vi "sub_peltier 1 control new.vi"(0 "Save File":path, 1 "Save Data to File":bool caption="Save?", 2 "Sample Rate (s)":i16=1, 9 "COM":i16, 12 "Array #":i32, 13 "Control Settings":T1={"Control Sensor Offset"=0.0, "Set Limit Low"=-20.0, "Set Limit High"=100.0, "Derivative Gain"=0.0, "Integral Gain"=0.0, "Proportional Bandwidth"=50.0}) -> ()   [LabVIEW 2021]
uses:
  <vilib>/Instr/_visa.llb/VISA Find Search Mode.ctl
  <vilib>/Utility/error.llb/DialogType.ctl
  globalvariables.vi
  <vilib>/Utility/file.llb/Write Delimited Spreadsheet (string).vi
  <vilib>/Utility/file.llb/Write Delimited Spreadsheet (DBL).vi
panel:
  in  "Controller Settings":enum32{"Page 1"}(tab)
  in  "Alarm Settings":enum32{"Page 1"}(tab)
  in  "Shutdown Output w/ Alarm 2":bool
  in  "Clear Alarm Latch":bool
  in  "Shutdown Output w/ Alarm 1":bool
  in  "Alarm 2 Deadband":dbl
  in  "Alarm 2 Low":dbl
  in  "Alarm 2 High":dbl=60.0
  in  "Alarm 1 Deadband":dbl
  in  "Alarm 1 Low":dbl
  in  "Alarm 1 High":dbl=60.0
  in  "Alarm Latch":T2(radio)
  out "Alarm":bool
  in  "Graph Data":enum32{"Tab 1"}(tab)
  out "Elapsed Time":dbl=-3262346310.140625
  out "Start Sample Time":timestamp=timestamp(3262346310.140625 s since 1904-01-01)
  out "Sample in Time":timestamp
  out "Set Temperature":dbl
  out "Input 2 Sensor":dbl
  out "Control Sensor":dbl
  in  "Misc Settings":enum32{"Page 1"}(tab)
  in  "Analog Output Multiplier":dbl=1.0
  in  "Sensor Type":enum32{"15K", "10K"}(radio)=enum."10K"
  in  "Output Polarity":enum32{"Cool", "Heat "}(radio)
  in  "EEPROM Write Enable":bool
  in  "Temperature 2 Display":T3(radio)=enum."Radio Selection 3"
  out "Firmware Version":string
  out "CRC Error":bool
  out "error out":errorcluster
  out "Reading Configuration":sgl
  in  "Display":enum32{"Page 1"}(tab)
  out "Power":i16(slide) scale=0.0..100.0
  out "Strip Chart":T4(graph)
  out "Sampling":bool
  in  "Run Peltier":bool
  # "%"
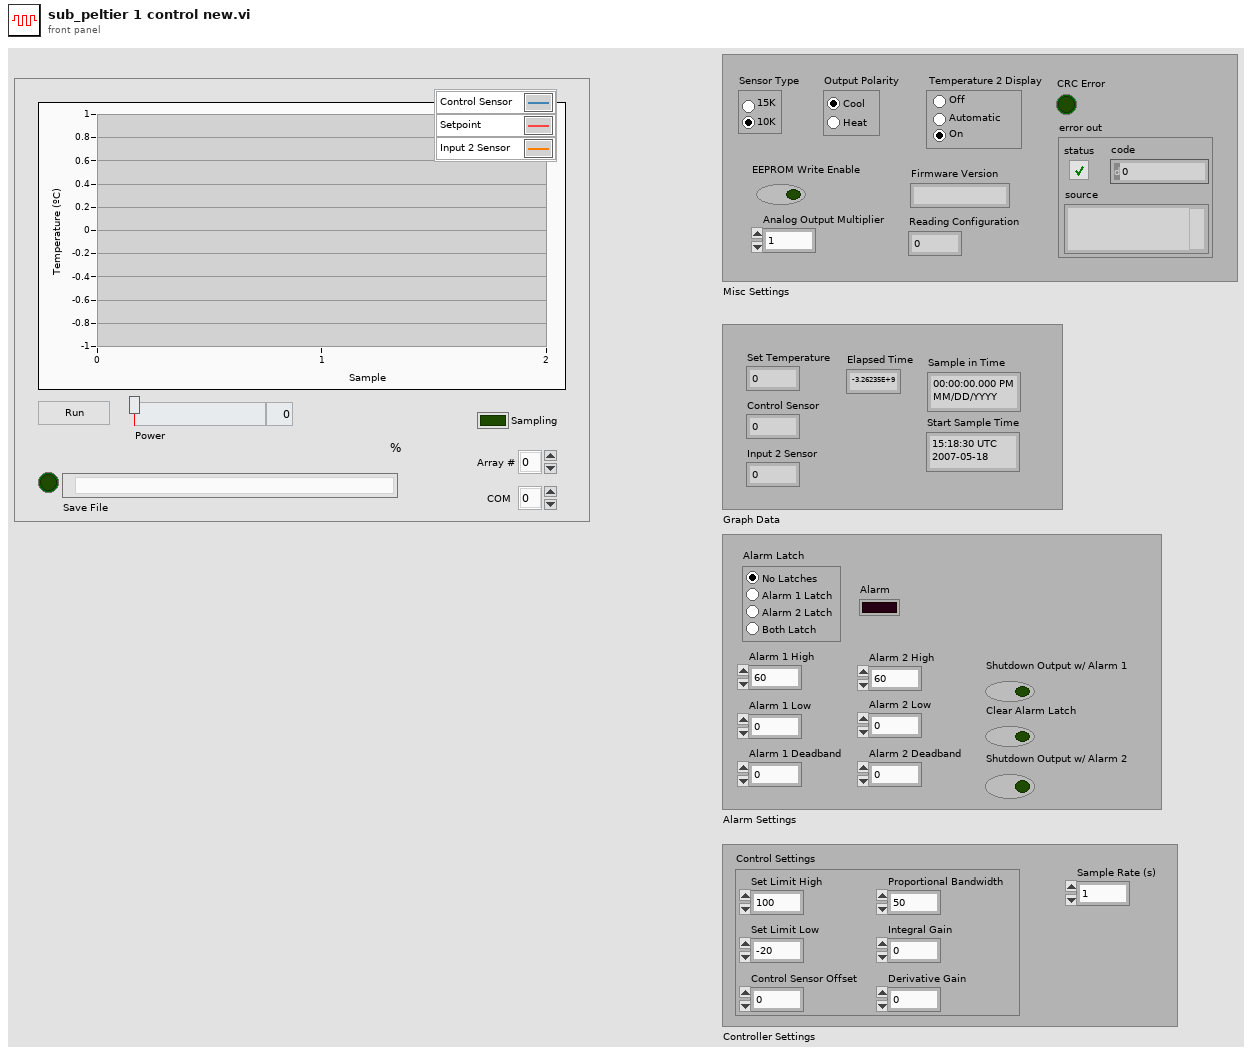
[diagram p1: front panel]
types:
  T1 = cluster{"Control Sensor Offset":dbl, "Set Limit Low":dbl, "Set Limit High":dbl, "Derivative Gain":dbl, "Integral Gain":dbl, "Proportional Bandwidth":dbl}
  T2 = enum32{"Radio Selection 1", "Radio Selection 2", "Radio Selection 3", "Radio Selection 4"}
  T3 = enum32{"Radio Selection 1", "Radio Selection 2", "Radio Selection 3"}
  T4 = cluster{"TEMPERATURE":dbl, "Value":dbl, "Value 2":dbl}
  T5 = cluster{"Read Model":bool, "Read Settings":bool, "End":bool, "CRC Error":bool, "Final Loop":bool}
  T6 = typedef "VISA Find Search Mode.ctl" = u32
  T7 = cluster{"TEMPERATURE":dbl, "Value":dbl, "Value 2":dbl}[]
  T8 = cluster{"SET POINT":dbl, "SET POINT":dbl, "SET POINT":dbl}
  T9 = typedef "DialogType.ctl" = u16
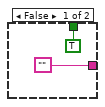
[diagram p2: hidden frame]
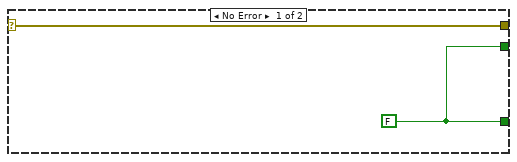
[diagram p3: hidden frame]
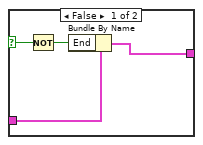
[diagram p11: hidden frame]
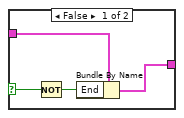
[diagram p13: hidden frame]
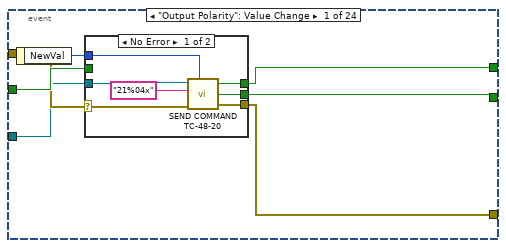
[diagram p14: hidden frame]
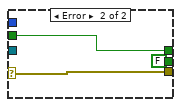
[diagram p15: hidden frame]
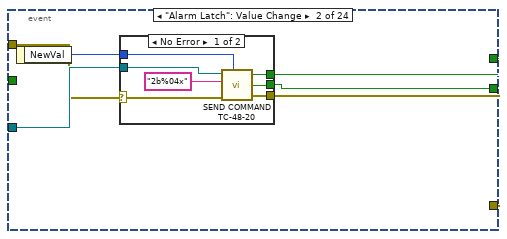
[diagram p16: hidden frame]
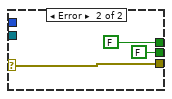
[diagram p17: hidden frame]
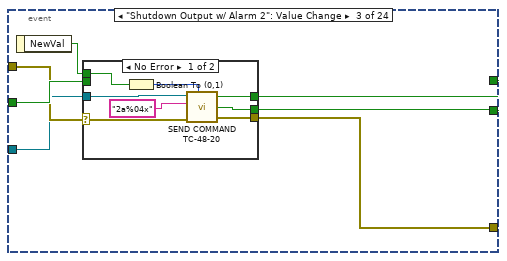
[diagram p18: hidden frame]
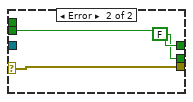
[diagram p19: hidden frame]
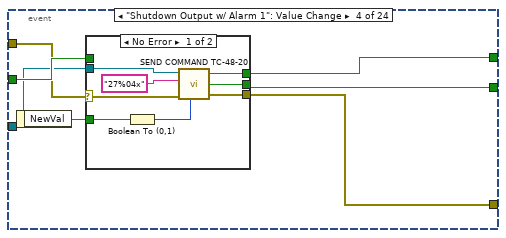
[diagram p20: hidden frame]
diagram:
  w1 = FALSE  # Final Loop
  w2 = FALSE  # CRC Error
  w3 = FALSE  # End
  w5 = TRUE  # Read Settings
  w6 = TRUE  # Read Model
  # "Connect to Peltier Controller"
  # "CHECK CONTROLS"
  n1 = Bundle("Read Model"=w6, "Read Settings"=w5, "End"=w3, "CRC Error"=w2, "Final Loop"=w1) -> (w4:T5)  [unwired: 1 in]
  n2 = while {
    tunnel: [w35] -> w10
    tunnel: [w30] -> w9
    tunnel: errorcluster {"status"=FALSE, "code"=0, "source"=""} ("Startup error in (no error)") -> [w34]
    tunnel: w4 -> [w28]
    tunnel: [w25] -> w8
    stop <- w29 continue-if-true
    w22 = u16 0 items=["None", "XON/XOFF", "RTS/CTS", "XON/XOFF & RTS/CTS", "DTR/DSR", "XON/XOFF & DTR/DSR"] ("Serial Settings:Flow Control")
    w18 = u16 0 items=["None", "Odd", "Even", "Mark", "Space"] ("Serial Settings:Parity")
    w23 = T6 4 items=["Canonical Names Only"=0, "Aliases Only"=1, "Include Matching Aliases"=2, "Include All Aliases"=4] ("Search Mode")
    n3 = Greater Than 0?(x="COM") -> (x > 0?=w13:bool)
    n4 = case shown="True" w13 {
      tunnel: "COM" -> [_ w44]
      tunnel: ["" w41] -> w11
      tunnel: [TRUE FALSE] -> w27
      frame False {
      }
      frame True {
        n5 = Number To Decimal String(number=w44) -> (decimal integer string=w42:string)  [unwired: 1 in]
        n6 = Concatenate Strings("COM", w42) -> (w41:string)
      }
    }
    n7 = property on="Firmware Version" class="Str"("Value"="") -> ()  [unwired: 2 in, 2 out]
    n8 = VISA Find Resource(8:w34, 10:w23) -> (0:w17:errorcluster)  [unwired: 1 in, 2 out]
    n9 = Coerce To Type(0:w11, 1:refnum<visa-resource-name> refnum ("SELECT PORT")) -> (2:w14:refnum<visa-resource-name>)
    n10 = property class="Instr" props=["Baud", "Data Bits", "Parity", "Stop Bits", "Flow Cntrl", "Rsrc Name", "Is Connected"](reference=w14, error in=w17, "Baud"=u32 115200 ("Numeric 6"), "Data Bits"=u16 8, "Parity"=w18, "Stop Bits"=u16 10, "Flow Cntrl"=w22) -> (reference out=w32:refnum<visa-resource-name>, error out=w33:errorcluster)  [unwired: 2 out]
    n11 = VISA Set I/O Buffer Size(VISA resource name=w32, error in (no error)=w33) -> (VISA resource name out=w36:refnum<visa-resource-name>, error out=w37:errorcluster)  [unwired: 2 in]
    n12 = VISA Flush I/O Buffer(VISA resource name=w36, error in (no error)=w37) -> (VISA resource name out=w35:refnum<visa-resource-name>, error out=w31:errorcluster)  [unwired: 1 in]
    n13 = case shown="Error" w31 {
      selector: w31 -> [w46 w50]
      tunnel: [w46 w50] -> w30
      tunnel: [w45 w48] -> w29
      tunnel: [w45 w47] -> w26
      frame No Error {
        w45 = FALSE
      }
      frame Error {
        n14 = Two Button Dialog(message=" Unable to communicate with controller (Error 1), check:\n• Controller is ON and correctly wired\n• Correct communications port is selected\n• Another program is not using the communications port ", 1:"EXIT" ("F button name (\"Cancel\")"), 2:"RESTART" ("T button name (\"OK\")")) -> (T button?=w49:bool)
        n15 = case shown="True" w49 {
          selector: w49 -> [w54 w55]
          tunnel: [w54 w55] -> w48
          frame False {
          }
          frame True {
            n16 = Wait (ms)(milliseconds to wait=u32 5000) -> ()  [unwired: 1 out]
          }
        }
        n17 = Not(x=w48) -> (.not. x?=w47:bool)
      }
    }
    n18 = Or(x=w27, y=w26) -> (x .or. y?=w24:bool)
    n19 = Bundle By Name(cluster=w28, "End"=w24) -> (w25:T5)
  }
  n20 = while {
    shift-right: [w64] -> _
    shift-left: w8 -> [w74]
    tunnel: w10 -> [w91]
    tunnel: w9 -> [w80]
    i -> [w65]
    stop <- w63 stop-if-true
    n21 = global read "globalvariables.vi" "Peltier Update"() -> (w78:bool[])
    n22 = property on="Array #" class="DigNum (strict)"() -> ("Value"=w76:i32)  [unwired: 2 in, 2 out]
    n23 = Bundle By Name(cluster=w74, "CRC Error"=FALSE) -> (w75:T5)
    n24 = Index Array(array=w78, index=w76) -> (element=w77:bool)
    n25 = case shown="True" w77 {
      tunnel: w75 -> [w105 w107]
      tunnel: [w105 w106] -> w60
      frame False {
      }
      frame True {
        n26 = global read "globalvariables.vi" "Peltier Set Temp"() -> (w115:dbl[])
        n27 = global read "globalvariables.vi" "Peltier Update"() -> (w113:bool[])
        n28 = global read "globalvariables.vi" "Peltier Stop"() -> (w108:bool)
        n29 = global read "globalvariables.vi" "Peltier Save"() -> (w109:bool)
        n30 = property on="Array #" class="DigNum (strict)"() -> ("Value"=w112:i32)  [unwired: 2 in, 2 out]
        n31 = case shown="True" w108 {
          selector: w108 -> [_ w118]
          tunnel: w107 -> [w116 w120]
          tunnel: [w116 w119] -> w106
          frame False {
          }
          frame True {
            n32 = Bundle By Name(cluster=w120, "End"=w118) -> (w119:T5)
            n33 = property on="Run Peltier" class="Bool (strict)"("Value"=FALSE ("Run Peltier")) -> ()  [unwired: 2 in, 2 out]
          }
        }
        n34 = property on="Save Data to File" class="Bool (strict)"("Value"=w109) -> ()  [unwired: 2 in, 2 out]
        n35 = Index Array(array=w115, index=w112) -> (element=w114:dbl)
        n36 = Replace Array Subset(array=w113, new element=FALSE ("Is Peltier Command Ready?"), index=w112) -> (w110:bool[])
        n37 = property on="Set Temperature" class="DigNum (strict)"("Val(Sgnl)"=w114) -> ()  [unwired: 2 in, 2 out]
        n38 = global write "globalvariables.vi" "Peltier Update"(w110) -> ()
      }
    }
    n39 = flat-sequence {
      tunnel: [w1168] -> w90
      tunnel: [w1167] -> w89
      tunnel: [w1166] -> w88
      tunnel: w60 -> [w1165]
      tunnel: w91 -> [w1164]
      tunnel: w80 -> [w1163]
      tunnel: w90 -> [w1288]
      tunnel: w89 -> [w1292]
      tunnel: w88 -> [w1291]
      tunnel: [w1290] -> w83
      tunnel: [w1289] -> w82
      tunnel: [w1287] -> w85
      frame #0 {
        n40 = case shown="No Error" w1163 {
          selector: w1163 -> [w1171 w1286]
          tunnel: [w1175 w1286] -> w1168
          tunnel: [w1174 w1285] -> w1167
          tunnel: [w1173 w1284] -> w1166
          tunnel: w1164 -> [w1172 w1285]
          tunnel: w1165 -> [w1170 w1284]
          frame No Error {
            n41 = Unbundle By Name(w1170) -> ("Read Model"=w1169:bool)
            n42 = case shown="True" w1169 {
              tunnel: [w1176 w1180] -> w1175
              tunnel: [w1177 w1182] -> w1174
              tunnel: w1170 -> [w1178 w1184]
              tunnel: [w1178 w1183] -> w1173
              tunnel: w1172 -> [w1177 w1182]
              tunnel: w1171 -> [w1176 w1179]
              frame False {
              }
              frame True {
                n43 = while {
                  tunnel: w1184 -> [w1188]
                  tunnel: [w1202] -> w1183
                  tunnel: w1182 -> [w1193]
                  tunnel: [w1194] -> w1180
                  tunnel: w1179 -> [w1190]
                  i -> [w1198]
                  stop <- w1196 stop-if-true
                  n44 = Greater Or Equal?(x=w1198, y=3) -> (x >= y?=w1197:bool)
                  n45 = call "QUERY MODEL9613.vi"("Communications Port"=w1193) -> ("error out"=w1191:errorcluster, "CRC ERROR"=w1186:bool, "CONTROLLER MODEL"=w1195:string)  [unwired: 3 in]
                  n46 = case shown="True" w1186 {
                    selector: w1186 -> [_ w1205]
                    tunnel: [w1203 w1206] -> w1187
                    tunnel: w1188 -> [w1203 w1204]
                    frame False {
                    }
                    frame True {
                      n47 = Bundle By Name(cluster=w1204, "CRC Error"=w1205) -> (w1206:T5)
                    }
                  }
                  n48 = case shown="True" w1197 {
                    tunnel: w1187 -> [w1208 w1212]
                    tunnel: [w1208 w1211] -> w1189
                    tunnel: [FALSE ("true") w1209] -> w1185
                    frame False {
                    }
                    frame True {
                      n49 = One Button Dialog(message="Commuincation Error") -> (true=w1209:bool)  [unwired: 1 in]
                      n50 = Bundle By Name(cluster=w1212, "End"=w1209) -> (w1211:T5)
                    }
                  }
                  n51 = Wait Until Next ms Multiple(millisecond multiple=u32 120) -> ()  [unwired: 1 out]
                  n52 = Equal?(x=w1195, y="9613") -> (x = y?=w1192:bool)
                  n53 = Merge Errors(w1190, w1191) -> (w1194:errorcluster)
                  n54 = Compound Arithmetic op=OR(w1192, w1186, w1185) -> (w1196:bool)
                  n55 = case shown="True" w1192 {
                    tunnel: [w1216 w1224] -> w1202
                    tunnel: w1193 -> [_ w1222]
                    tunnel: w1189 -> [w1213 w1218]
                    frame False {
                      n56 = Bundle By Name(cluster=w1213, "Read Model"=TRUE, "Read Settings"=FALSE) -> (w1216:T5)
                    }
                    frame True {
                      n57 = call "QUERY FIRMWARE VERSION M9613.vi"("Communications Port"=w1222) -> ("error out"=w1221:errorcluster, "VERSION NUMBER"=w1220:u32)  [unwired: 8 in, 1 out]
                      n58 = Bundle By Name(cluster=w1218, "Read Model"=FALSE) -> (w1224:T5)
                      n59 = case shown="No Error" w1221 {
                        tunnel: w1220 -> [w1227 _]
                        tunnel: [w1226 ""] -> w1219
                        tunnel: [w1225 2] -> w1217
                        frame No Error {
                          n60 = case shown="0, Default" w1227 {
                            tunnel: ["B" "C" "D" "E" "F" "G" "H" "I" "J" "K" "L" "M" "N" "O" "P" "Q" "R" "S" "T" "U" "V" "W" "X" "Y" "Z" "" "A"] -> w1226
                            tunnel: [2 2 2 2 2 2 0 0 0 0 0 0 0 0 0 0 0 0 0 0 0 0 0 0 0 2 2] -> w1225
                            frame 2 {
                            }
                            frame 3 {
                            }
                            frame 4 {
                            }
                            frame 5 {
                            }
                            frame 6 {
                            }
                            frame 7 {
                            }
                            frame 8 {
                            }
                            frame 9 {
                            }
                            frame 10 {
                            }
                            frame 11 {
                            }
                            frame 12 {
                            }
                            frame 13 {
                            }
                            frame 14 {
                            }
                            frame 15 {
                            }
                            frame 16 {
                            }
                            frame 17 {
                            }
                            frame 18 {
                            }
                            frame 19 {
                            }
                            frame 20 {
                            }
                            frame 21 {
                            }
                            frame 22 {
                            }
                            frame 23 {
                            }
                            frame 24 {
                            }
                            frame 25 {
                            }
                            frame 26 {
                            }
                            frame 0, Default {
                            }
                            frame 1 {
                            }
                          }
                        }
                        frame Error {
                        }
                      }
                      "Firmware Version" <- w1219
                      n61 = property on="EEPROM Write Enable" class="Bool (strict)"("Disabled"=w1217) -> ()  [unwired: 2 in, 2 out]
                    }
                  }
                }
                n62 = property on="Strip Chart" class="WFChart (strict)"("History Data"=T7 []) -> ()  [unwired: 2 in, 2 out]
              }
            }
          }
          frame Error {
          }
        }
      }
      frame #1 {
        n63 = case shown="No Error" w1288 {
          selector: w1288 -> [w1295 w1494]
          tunnel: w1292 -> [w1299 w1495]
          tunnel: w1291 -> [w1293 w1498]
          tunnel: [w1298 w1497] -> w1290
          tunnel: [w1297 w1494] -> w1289
          tunnel: [w1296 w1495] -> w1287
          frame No Error {
            n64 = Unbundle By Name(w1293) -> ("Read Settings"=w1294:bool)
            n65 = case shown="True" w1294 {
              tunnel: w1295 -> [w1302 w1312]
              tunnel: w1299 -> [w1300 w1309]
              tunnel: w1293 -> [w1303 w1306]
              tunnel: [w1303 w1311] -> w1298
              tunnel: [w1302 w1310] -> w1297
              tunnel: [w1300 w1308] -> w1296
              frame False {
                n66 = property on="Reading Configuration" class="DigNum (strict)"("Value"=0) -> ()  [unwired: 2 in, 2 out]
              }
              frame True {
                n67 = for {
                  N: 21 -> [_]
                  tunnel: w1309 -> [w1322]
                  tunnel: w1312 -> [w1328]
                  tunnel: [w1321] -> w1310
                  tunnel: [w1322] -> w1308
                  tunnel: w1306 -> [w1318]
                  tunnel: [w1315] -> w1305
                  i -> [w1313]
                  n68 = Divide(x=w1313, y=21) -> (x/y=w1327:dbl)
                  n69 = case shown="8" w1313 {
                    tunnel: w1322 -> [w1343 w1348 w1356 w1362 w1369 w1373 w1383 w1391 w1407 w1412 w1419 w1425 w1433 w1443 w1455 w1459 w1467 w1472 w1479 w1487 w1491]
                    tunnel: w1328 -> [w1339 w1347 w1353 w1360 w1368 w1372 w1382 w1386 w1406 w1410 w1416 w1422 w1428 w1442 w1454 w1461 w1465 w1473 w1478 w1486 w1492]
                    tunnel: [w1342 _ _ _ w1365 _ _ _ _ _ _ _ _ _ _ _ _ _ _ _ _] -> w1319
                    tunnel: [FALSE ("CRC") w1344 w1351 w1358 FALSE ("CRC") w1370 w1377 w1385 w1395 w1408 w1415 w1421 w1426 w1436 w1448 w1457 w1463 w1468 w1474 w1480 w1489] -> w1317
                    tunnel: [w1341 w1346 w1355 w1361 w1367 w1374 w1381 w1390 w1400 w1411 w1418 w1424 w1432 w1440 w1452 w1460 w1466 w1470 w1477 w1485 w1493] -> w1323
                    tunnel: [w1338 w1345 w1352 w1357 w1364 w1371 w1376 w1384 w1396 w1409 w1414 w1420 w1427 w1437 w1449 w1456 w1462 w1469 w1475 w1481 w1488] -> w1316
                    frame 0, Default {
                      n70 = property on="Power" class="Slide (strict)"() -> ("Value"=w1342:i16)  [unwired: 2 in, 2 out]
                      n71 = call "QUERY INPUT 1 M9613.vi"("Communications Port"=w1343, "error in"=w1339) -> ("CRC ERROR"=w1338:bool, "TEMPERATURE"=w1340:dbl, "error out"=w1341:errorcluster)
                      n72 = property on="Control Sensor" class="DigNum (strict)"("Value"=w1340) -> ()  [unwired: 2 in, 2 out]
                    }
                    frame 1 {
                      n73 = call "QUERY ALARMS M9613.vi"("Communications Port"=w1348, "error in"=w1347) -> ("CRC ERROR"=w1345:bool, "End"=w1344:bool, "ALARM VALUE"=w1349:dbl, "error out"=w1346:errorcluster)
                      n74 = Not Equal To 0?(x=w1349) -> (x != 0?=→"Alarm":bool)
                    }
                    frame 2 {
                      n75 = call "QUERY CONTROL MODE M9613.vi"("Communications Port"=w1356, "error in"=w1353) -> ("CRC ERROR"=w1352:bool, "End"=w1351:bool, "CONTROL MODE"=w1354:dbl, "error out"=w1355:errorcluster)
                      n76 = property on="Output Polarity" class="RadioBtnsControl (strict)"("Value"=w1354) -> ()  [unwired: 2 in, 2 out]
                    }
                    frame 3 {
                      n77 = call "QUERY ALARM LATCH SETTING M9613.vi"("Communications Port"=w1362, "error in"=w1360) -> ("CRC ERROR"=w1357:bool, "End"=w1358:bool, "ALARM LATCH SETTING"=w1359:dbl, "error out"=w1361:errorcluster)
                      n78 = property on="Alarm Latch" class="RadioBtnsControl (strict)"("Value"=w1359) -> ()  [unwired: 2 in, 2 out]
                    }
                    frame 4 {
                      n79 = call "QUERY POWER OUT M9613.vi"("Communications Port"=w1369, "error in"=w1368) -> ("CRC ERROR"=w1364:bool, "POWER OUT, %"=w1366:dbl, "error out"=w1367:errorcluster)
                      n80 = To Word Integer(number=w1366) -> (16bit integer=w1365:i16)
                    }
                    frame 5 {
                      n81 = call "QUERY SETPOINT M9613.vi"("Communications Port"=w1373, "error in"=w1372) -> ("CRC ERROR"=w1371:bool, "End"=w1370:bool, "SET POINT"=w1375:dbl, "error out"=w1374:errorcluster)
                      n82 = property on="Set Temperature" class="DigNum (strict)"("Value"=w1375) -> ()  [unwired: 2 in, 2 out]
                    }
                    frame 6 {
                      n83 = call "QUERY ALARM 2 STATUS M9613.vi"("Communications Port"=w1383, "error in"=w1382) -> ("CRC ERROR"=w1376:bool, "End"=w1377:bool, "ALARM 2 OUTPUT STATUS"=w1378:dbl, "error out"=w1381:errorcluster)
                      n84 = Number To Boolean Array(number=w1378) -> (Boolean array=w1380:bool[])
                      n85 = Or Array Elements(Boolean array=w1380) -> (logical OR=w1379:bool)
                      n86 = property on="Shutdown Output w/ Alarm 2" class="Bool (strict)"("Value"=w1379) -> ()  [unwired: 2 in, 2 out]
                    }
                    frame 7 {
                      n87 = call "QUERY ALARM 1 STATUS M9613.vi"("Communications Port"=w1391, "error in"=w1386) -> ("CRC ERROR"=w1384:bool, "End"=w1385:bool, "ALARM 2 OUTPUT STATUS"=w1389:dbl, "error out"=w1390:errorcluster)
                      n88 = Number To Boolean Array(number=w1389) -> (Boolean array=w1388:bool[])
                      n89 = Or Array Elements(Boolean array=w1388) -> (logical OR=w1387:bool)
                      n90 = property on="Shutdown Output w/ Alarm 1" class="Bool (strict)"("Value"=w1387) -> ()  [unwired: 2 in, 2 out]
                    }
                    frame 8 {
                      n91 = call "QUERY PROPORTIONAL BW M9613.vi"("Communications Port"=w1407, "error in"=w1406) -> ("CRC ERROR"=w1399:bool, "End"=w1394:bool, "PROPOTIONAL BW"=w1403:dbl, "error out"=w1402:errorcluster)
                      n92 = call "QUERY INTEGRAL GAIN M9613.vi"("Communications Port"=w1407, "error in"=w1402) -> ("CRC ERROR"=w1398:bool, "End"=w1393:bool, "INTEGRAL GAIN"=w1404:dbl, "error out"=w1401:errorcluster)
                      n93 = call "QUERY DERIVATIVE GAIN M9613.vi"("Communications Port"=w1407, "error in"=w1401) -> ("CRC ERROR"=w1397:bool, "End"=w1392:bool, "DERIVATIVE GAIN"=w1405:dbl, "error out"=w1400:errorcluster)
                      n94 = property on="Proportional Bandwidth" class="DigNum (strict)"("Value"=w1403) -> ()  [unwired: 2 in, 2 out]
                      n95 = property on="Integral Gain" class="DigNum (strict)"("Value"=w1404) -> ()  [unwired: 2 in, 2 out]
                      n96 = property on="Derivative Gain" class="DigNum (strict)"("Value"=w1405) -> ()  [unwired: 2 in, 2 out]
                      n97 = Compound Arithmetic op=OR(w1399, w1398, w1397) -> (w1396:bool)
                      n98 = Compound Arithmetic op=OR(w1394, w1393, w1392) -> (w1395:bool)
                    }
                    frame 9 {
                      n99 = call "INPUT 1 SENSOR OFFSET M9613.vi"("Communications Port"=w1412, "error in"=w1410) -> ("CRC ERROR"=w1409:bool, "End"=w1408:bool, "INPUT 1 SENSOR OFFSET"=w1413:dbl, "error out"=w1411:errorcluster)
                      n100 = property on="Control Sensor Offset" class="DigNum (strict)"("Value"=w1413) -> ()  [unwired: 2 in, 2 out]
                    }
                    frame 10 {
                      n101 = call "QUERY ALARM LATCH SETTING M9613.vi"("Communications Port"=w1419, "error in"=w1416) -> ("CRC ERROR"=w1414:bool, "End"=w1415:bool, "ALARM LATCH SETTING"=w1417:dbl, "error out"=w1418:errorcluster)
                      n102 = property on="Alarm Latch" class="RadioBtnsControl (strict)"("Value"=w1417) -> ()  [unwired: 2 in, 2 out]
                    }
                    frame 11 {
                      n103 = call "QUERY SENSOR TYPE M9613.vi"("Communications Port"=w1425, "error in"=w1422) -> ("CRC ERROR"=w1420:bool, "End"=w1421:bool, "SENSOR TYPE"=w1423:dbl, "error out"=w1424:errorcluster)
                      n104 = property on="Sensor Type" class="RadioBtnsControl (strict)"("Value"=w1423) -> ()  [unwired: 2 in, 2 out]
                    }
                    frame 12 {
                      n105 = call "QUERY ALARM 1 DEADBAND M9613.vi"("Communications Port"=w1433, "error in"=w1428) -> ("CRC ERROR"=w1427:bool, "End"=w1426:bool, "ALARM 1 DEADBAND"=w1430:dbl, "error out"=w1432:errorcluster)
                      n106 = Divide(x=w1430, y=10.0) -> (x/y=w1431:dbl)
                      n107 = property on="Alarm 1 Deadband" class="DigNum (strict)"("Value"=w1431) -> ()  [unwired: 2 in, 2 out]
                    }
                    frame 13 {
                      n108 = call "QUERY HIGH ALARM SET POINT M9613.vi"("Communications Port"=w1443, "error in"=w1442) -> ("CRC ERROR"=w1435:bool, "HIGH ALARM SETPOINT INPUT 1"=w1438:dbl, "error out"=w1441:errorcluster)
                      n109 = call "QUERY LOW ALARM SET POINT M9613.vi"("Communications Port"=w1443, "error in"=w1441) -> ("CRC ERROR"=w1434:bool, "End"=w1436:bool, "LOW ALARM SETPOINT"=w1439:dbl, "error out"=w1440:errorcluster)
                      n110 = Or(x=w1435, y=w1434) -> (x .or. y?=w1437:bool)
                      n111 = property on="Alarm 1 High" class="DigNum (strict)"("Value"=w1438) -> ()  [unwired: 2 in, 2 out]
                      n112 = property on="Alarm 1 Low" class="DigNum (strict)"("Value"=w1439) -> ()  [unwired: 2 in, 2 out]
                    }
                    frame 14 {
                      n113 = call "QUERY HIGH ALARM SET POINT INPUT 2 M9613.vi"("Communications Port"=w1455, "error in"=w1454) -> ("CRC ERROR"=w1447:bool, "End"=w1446:bool, "HIGH ALARM SETPOINT INPUT 2"=w1451:dbl, "error out"=w1453:errorcluster)
                      n114 = call "QUERY LOW ALARM SET POINT INPUT 2 M9613.vi"("Communications Port"=w1455, "error in"=w1453) -> ("CRC ERROR"=w1445:bool, "End"=w1444:bool, "LOW ALARM SETPOINT INPUT 2"=w1450:dbl, "error out"=w1452:errorcluster)
                      n115 = Or(x=w1447, y=w1445) -> (x .or. y?=w1449:bool)
                      n116 = Or(x=w1446, y=w1444) -> (x .or. y?=w1448:bool)
                      n117 = property on="Alarm 2 High" class="DigNum (strict)"("Value"=w1451) -> ()  [unwired: 2 in, 2 out]
                      n118 = property on="Alarm 2 Low" class="DigNum (strict)"("Value"=w1450) -> ()  [unwired: 2 in, 2 out]
                    }
                    frame 15 {
                      n119 = call "QUERY ANALOG OUTPUT MULTIPLIER M9613.vi"("Communications Port"=w1459, "error in"=w1461) -> ("CRC ERROR"=w1456:bool, "End"=w1457:bool, "ANALOG OUTPUT MULTIPLIER"=w1458:dbl, "error out"=w1460:errorcluster)
                      n120 = property on="Analog Output Multiplier" class="DigNum (strict)"("Value"=w1458) -> ()  [unwired: 2 in, 2 out]
                    }
                    frame 16 {
                      n121 = call "QUERY TEMP 2 DISPLAY M9613.vi"("Communications Port"=w1467, "error in"=w1465) -> ("CRC ERROR"=w1462:bool, "End"=w1463:bool, "TEMPERATURE 2 DISPLAY"=w1464:dbl, "error out"=w1466:errorcluster)
                      n122 = property on="Temperature 2 Display" class="RadioBtnsControl (strict)"("Value"=w1464) -> ()  [unwired: 2 in, 2 out]
                    }
                    frame 17 {
                      n123 = call "QUERY LOW SET RANGE M9613.vi"("Communications Port"=w1472, "error in"=w1473) -> ("CRC ERROR"=w1469:bool, "End"=w1468:bool, "LOW SET RANGE"=w1471:dbl, "error out"=w1470:errorcluster)
                      n124 = property on="Set Limit Low" class="DigNum (strict)"("Value"=w1471) -> ()  [unwired: 2 in, 2 out]
                    }
                    frame 18 {
                      n125 = call "QUERY HIGH SET RANGE M9613.vi"("Communications Port"=w1479, "error in"=w1478) -> ("CRC ERROR"=w1475:bool, "End"=w1474:bool, "HIGH SET RANGE"=w1476:dbl, "error out"=w1477:errorcluster)
                      n126 = property on="Set Limit High" class="DigNum (strict)"("Value"=w1476) -> ()  [unwired: 2 in, 2 out]
                    }
                    frame 19 {
                      n127 = call "QUERY OUTPUT ON M9613.vi"("Communications Port"=w1487, "error in"=w1486) -> ("CRC ERROR"=w1481:bool, "End"=w1480:bool, "OUTPUT ENABLE"=w1484:i8, "error out"=w1485:errorcluster)
                      n128 = Number To Boolean Array(number=w1484) -> (Boolean array=w1483:bool[])
                      n129 = Or Array Elements(Boolean array=w1483) -> (logical OR=w1482:bool)
                      n130 = property on="Run Peltier" class="Bool (strict)"("Value"=w1482) -> ()  [unwired: 2 in, 2 out]
                    }
                    frame 20 {
                      n131 = call "QUERY EEPROM WRITE ENABLE.vi"("Communications Port"=w1491, "error IO"=w1492) -> ("EEPROM WRITE\nENABLED"=w1490:bool, "End"=w1489:bool, "CRC"=w1488:bool, "error IO 2"=w1493:errorcluster)
                      n132 = property on="EEPROM Write Enable" class="Bool (strict)"("Value"=w1490) -> ()  [unwired: 2 in, 2 out]
                    }
                  }
                  "Power" <- w1319
                  n133 = Multiply(x=100, y=w1327) -> (x*y=→"Reading Configuration":dbl)
                  n134 = case shown="True" w1317 {
                    selector: w1317 -> [_ w1331]
                    tunnel: w1318 -> [w1329 w1332]
                    tunnel: [w1329 w1330] -> w1314
                    frame False {
                    }
                    frame True {
                      n135 = Bundle By Name(cluster=w1332, "End"=w1331) -> (w1330:T5)
                    }
                  }
                  n136 = case shown="True" w1316 {
                    selector: w1316 -> [_ w1336]
                    tunnel: w1314 -> [w1333 w1334]
                    tunnel: [w1333 w1335] -> w1315
                    tunnel: [w1333 w1334] -> _
                    frame False {
                    }
                    frame True {
                      n137 = Bundle By Name(cluster=w1334, "CRC Error"=w1336) -> (w1335:T5)
                    }
                  }
                  n138 = call <vilib>:"Simple Error Handler.vi"("error source (\" \")"="ERROR IN READ CONFIGURATION" ("error source (\" \")"), "error in (no error)"=w1323) -> ("error out"=w1321:errorcluster)  [unwired: 3 in, 4 out]
                }
                n139 = Bundle By Name(cluster=w1305, "Read Settings"=FALSE) -> (w1311:T5)
              }
            }
          }
          frame Error {
            w1496 = TRUE
            n140 = Bundle By Name(cluster=w1498, "Read Model"=w1496, "Read Settings"=w1496) -> (w1497:T5)
          }
        }
      }
    }
    n141 = case shown="Error" w82 {
      selector: w82 -> [w121 w123]
      tunnel: w83 -> [w122 w126]
      tunnel: [w122 w125] -> w58
      tunnel: [w121 w123] -> w81
      frame No Error {
      }
      frame Error {
        n142 = Two Button Dialog(message=" Unable to communicate with controller (Error 2), check:\n• Controller is ON and correctly wired\n• Correct communications port is selected\n• Another program is not using the communications port ", 1:"EXIT" ("F button name (\"Cancel\")"), 2:"RESTART" ("T button name (\"OK\")")) -> (T button?=w124:bool)
        n143 = case shown="True" w124 {
          selector: w124 -> [w133 _]
          tunnel: w126 -> [w132 w134]
          tunnel: [w130 w136] -> w125
          frame False {
            n144 = Not(x=w133) -> (.not. x?=w131:bool)
            n145 = Bundle By Name(cluster=w132, "End"=w131) -> (w130:T5)
          }
          frame True {
            w135 = TRUE
            n146 = Bundle By Name(cluster=w134, "Read Model"=w135, "Read Settings"=w135) -> (w136:T5)
          }
        }
      }
    }
    n147 = Unbundle By Name(w58) -> ("End"=w59:bool)
    n148 = case shown="True" w59 {
      tunnel: w58 -> [w92 w95]
      tunnel: [w92 w94] -> w57
      frame False {
      }
      frame True {
        n149 = property on="Run Peltier" class="Bool (strict)"("Value"=FALSE ("Run Peltier")) -> ()  [unwired: 2 in, 2 out]
        n150 = Bundle By Name(cluster=w95, "Final Loop"=TRUE ("Final loop")) -> (w94:T5)
      }
    }
    n151 = case shown="No Error" w81 {
      selector: w81 -> [w896 w1147]
      tunnel: [w900 w1147] -> w86
      tunnel: w85 -> [w899 _]
      tunnel: w57 -> [w898 w1148]
      tunnel: [w897 w1148] -> w87
      tunnel: w65 -> [w892 _]
      frame No Error {
        n152 = flat-sequence {
          tunnel: w896 -> [w919]
          tunnel: w899 -> [w917]
          tunnel: [w918] -> w912
          tunnel: [w916] -> w913
          tunnel: w898 -> [w915]
          tunnel: [w914] -> w911
          tunnel: [w952] -> w910
          tunnel: [w964] -> w909
          tunnel: w913 -> [w963]
          tunnel: w912 -> [w959]
          tunnel: w911 -> [w958]
          tunnel: [w956] -> w908
          tunnel: [w953] -> w893
          tunnel: w910 -> [w1038]
          tunnel: w909 -> [w1037]
          tunnel: [w1036] -> w907
          tunnel: [w1035] -> w906
          tunnel: [w1032] -> w905
          tunnel: w908 -> [w1034]
          tunnel: [w1034] -> w904
          tunnel: [w1033] -> w894
          tunnel: w893 -> [w1032]
          tunnel: [w1071] -> w903
          tunnel: [w1065] -> w902
          tunnel: [w1069] -> w901
          tunnel: [w1068] -> w895
          tunnel: w894 -> [w1068]
          tunnel: w904 -> [w1062]
          tunnel: w905 -> [w1066]
          tunnel: w906 -> [w1063]
          tunnel: w907 -> [w1064]
          tunnel: [w1102] -> w900
          tunnel: w903 -> [w1105]
          tunnel: w902 -> [w1093]
          tunnel: w901 -> [w1091]
          tunnel: [w1103] -> w897
          tunnel: w895 -> [w1097]
          tunnel: w892 -> [w1099]
          frame #0 {
            n153 = case shown="No Error" w919 {
              selector: w919 -> [w937 w950]
              tunnel: [w929 w950] -> w918
              tunnel: w917 -> [w930 w949]
              tunnel: [w930 w949] -> w916
              tunnel: w915 -> [w925 w948]
              tunnel: [w920 w946] -> w914
              frame No Error {
                # "CHECK ALARM STATUS"
                n154 = call "QUERY ALARMS M9613.vi"("Communications Port"=w930, "error in"=w937) -> ("CRC ERROR"=w927:bool, "End"=w923:bool, "ALARM VALUE"=w932:dbl, "error out"=w936:errorcluster)
                n155 = case shown="True" w923 {
                  selector: w923 -> [_ w940]
                  tunnel: w925 -> [w938 w941]
                  tunnel: [w938 w939] -> w924
                  frame False {
                  }
                  frame True {
                    n156 = Bundle By Name(cluster=w941, "End"=w940) -> (w939:T5)
                  }
                }
                n157 = call "DECODE ALARM STATUS TC4820.vi"("error in (no error)"=w936, "ALARM STATUS IN"=w932) -> ("error out"=w935:errorcluster, "READ CONTROLLER"=w921:bool)  [unwired: 1 in, 1 out]
                n158 = In Range and Coerce(upper limit=32, x=w932, lower limit=1) -> (In Range?=w931:bool)  [unwired: 1 out]
                n159 = call "QUERY ALARM SETPOINT DIABLE M9613.vi"("Communications Port"=w930, "error in"=w935) -> ("CRC Error"=w928:bool, "error out"=w929:errorcluster)  [unwired: 1 out]
                n160 = property on="Alarm" class="Bool (strict)"("Value"=w931, "Blinking"=w931) -> ()  [unwired: 2 in, 2 out]
                n161 = Or(x=w928, y=w927) -> (x .or. y?=w926:bool)
                n162 = case shown="True" w926 {
                  selector: w926 -> [_ w944]
                  tunnel: w924 -> [w942 w945]
                  tunnel: [w942 w943] -> w922
                  frame False {
                  }
                  frame True {
                    n163 = Bundle By Name(cluster=w945, "CRC Error"=w944) -> (w943:T5)
                  }
                }
                n164 = Bundle By Name(cluster=w922, "Read Settings"=w921) -> (w920:T5)
              }
              frame Error {
                n165 = Bundle By Name(cluster=w948, "Read Settings"=FALSE) -> (w946:T5)
              }
            }
          }
          frame #1 {
            # "READ TEMPERATURE"
            n166 = case shown="No Error" w959 {
              selector: w959 -> [w975 w1013]
              tunnel: w963 -> [w973 w1012]
              tunnel: [w979 w1013] -> w961
              tunnel: [w977 0.0] -> w954
              tunnel: [w973 w1012] -> w962
              tunnel: w958 -> [w970 w1011]
              tunnel: [w971 w1011] -> w957
              tunnel: [w965 -inf] -> w951
              frame No Error {
                n167 = call "QUERY SETPOINT M9613.vi"("Communications Port"=w973, "error in"=w975) -> ("CRC ERROR"=w976:bool, "End"=w966:bool, "SET POINT"=w965:dbl, "error out"=w980:errorcluster)
                n168 = property on="Set Temperature" class="DigNum (strict)"("Value"=w965) -> ()  [unwired: 2 in, 2 out]
                n169 = case shown="\"Radio Selection 3\"" "Temperature 2 Display" {
                  tunnel: w973 -> [_ w995 w1007]
                  tunnel: w980 -> [w992 w1000 w1006]
                  tunnel: [w992 w999 w1005] -> w979
                  tunnel: [w990 w994 w1002] -> w977
                  tunnel: [w989 w997 w1004] -> w974
                  tunnel: [w989 w993 w1001] -> w967
                  frame "Radio Selection 1", Default {
                    w990 = 0.0 ("TEMP. SENSOR 2")
                    w989 = FALSE
                    n170 = property on="Input 2 Sensor" class="DigNum (strict)"("Disabled"=2, "Value"=w990) -> ()  [unwired: 2 in, 2 out]
                  }
                  frame "Radio Selection 2" {
                    n171 = call "QUERY INPUT 2 M9613.vi"("Communications Port"=w995, "error in"=w1000) -> ("CRC ERROR"=w997:bool, "End"=w993:bool, "SECONDARY SENSOR VALUE"=w994:dbl, "error out"=w999:errorcluster)
                    "Input 2 Sensor" <- w994
                    n172 = property on="Input 2 Sensor" class="DigNum (strict)"("Disabled"=u8 0) -> ()  [unwired: 2 in, 2 out]
                    n173 = Wait Until Next ms Multiple(millisecond multiple=50) -> ()  [unwired: 1 out]
                  }
                  frame "Radio Selection 3" {
                    n174 = call "QUERY INPUT 2 M9613.vi"("Communications Port"=w1007, "error in"=w1006) -> ("CRC ERROR"=w1004:bool, "End"=w1001:bool, "SECONDARY SENSOR VALUE"=w1002:dbl, "error out"=w1005:errorcluster)
                    n175 = property on="Input 2 Sensor" class="DigNum (strict)"("Value"=w1002, "Disabled"=0) -> ()  [unwired: 2 in, 2 out]
                    n176 = Wait Until Next ms Multiple(millisecond multiple=u32 50) -> ()  [unwired: 1 out]
                  }
                }
                n177 = Or(x=w974, y=w976) -> (x .or. y?=w972:bool)
                n178 = Or(x=w967, y=w966) -> (x .or. y?=w968:bool)
                n179 = case shown="True" w968 {
                  selector: w968 -> [_ w983]
                  tunnel: w970 -> [w981 w984]
                  tunnel: [w981 w982] -> w969
                  frame False {
                  }
                  frame True {
                    n180 = Bundle By Name(cluster=w984, "End"=w983) -> (w982:T5)
                  }
                }
                n181 = case shown="True" w972 {
                  selector: w972 -> [_ w987]
                  tunnel: w969 -> [w985 w988]
                  tunnel: [w985 w986] -> w971
                  frame False {
                  }
                  frame True {
                    n182 = Bundle By Name(cluster=w988, "CRC Error"=w987) -> (w986:T5)
                  }
                }
              }
              frame Error {
              }
            }
            n183 = case shown="No Error" w961 {
              selector: w961 -> [w1021 w1031]
              tunnel: w962 -> [w1023 w1029]
              tunnel: [w1022 w1031] -> w952
              tunnel: [w1020 -inf] -> w955
              tunnel: [w1023 w1029] -> w964
              tunnel: w957 -> [w1016 w1028]
              tunnel: [w1014 w1028] -> w956
              frame No Error {
                n184 = global read "globalvariables.vi" "Peltier Control Sensor"() -> (w1019:dbl[])
                n185 = call "QUERY INPUT 1 M9613.vi"("Communications Port"=w1023, "error in"=w1021) -> ("CRC ERROR"=w1015:bool, "TEMPERATURE"=w1020:dbl, "error out"=w1022:errorcluster)
                "Control Sensor" <- w1020
                n186 = property on="Array #" class="DigNum (strict)"() -> ("Value"=w1017:i32)  [unwired: 2 in, 2 out]
                n187 = case shown="True" w1015 {
                  selector: w1015 -> [_ w1026]
                  tunnel: w1016 -> [w1024 w1027]
                  tunnel: [w1024 w1025] -> w1014
                  frame False {
                  }
                  frame True {
                    n188 = Bundle By Name(cluster=w1027, "CRC Error"=w1026) -> (w1025:T5)
                  }
                }
                n189 = Replace Array Subset(array=w1019, new element=w1020, index=w1017) -> (w1018:dbl[])
                n190 = global write "globalvariables.vi" "Peltier Control Sensor"(w1018) -> ()
              }
              frame Error {
              }
            }
            n191 = property on="Sampling" class="Bool (strict)"("Value"=TRUE) -> ()  [unwired: 2 in, 2 out]
            n192 = Build Array(w955, w954, w951) -> (w953:dbl[])
          }
          frame #2 {
            n193 = case shown="No Error" w1038 {
              selector: w1038 -> [w1046 w1061]
              tunnel: [w1046 w1061] -> w1036
              tunnel: w1037 -> [w1047 w1060]
              tunnel: [w1047 w1060] -> w1035
              tunnel: w1032 -> [w1045 _]
              frame No Error {
                n194 = local read "Temperature 2 Display"() -> (w1041:T3)
                n195 = property on="Strip Chart" class="WFChart (strict)"("YScale.Maximum"=8.0, "YScale.Minimum"=30.0) -> ()  [unwired: 2 in, 2 out]
                n196 = case shown="\"Radio Selection 1\", Default" w1041 {
                  tunnel: [w1052 w1058] -> w1042
                  tunnel: w1045 -> [w1049 w1057]
                  tunnel: [2 3] -> w1044
                  frame "Radio Selection 1", Default {
                    n197 = Index Array(array=w1049) -> (element #1=w1050:dbl, element #3=w1048:dbl)  [unwired: 3 in, 1 out]
                    n198 = Bundle(cluster=T4 {"TEMPERATURE"=0.0, "Value"=0.0, "Value 2"=0.0}, "TEMPERATURE"=w1050, "Value"=w1048) -> (w1052:T4)  [unwired: 1 in]
                  }
                  frame "Radio Selection 2", "Radio Selection 3" {
                    n199 = Index Array(array=w1057) -> (element #1=w1056:dbl, element #2=w1055:dbl, element #3=w1054:dbl)  [unwired: 3 in]
                    n200 = Bundle("SET POINT"=w1056, "SET POINT"=w1054, "SET POINT"=w1055) -> (w1058:T8)  [unwired: 1 in]
                  }
                }
                "Strip Chart" <- w1042
                n201 = property on="Strip Chart" class="WFChart (strict)"("LegPlots"=w1044, "YScale.UnitLabel.Text"="CELSIUS" ("Y Scale.Unit Label.Text")) -> ()  [unwired: 2 in, 2 out]
              }
              frame Error {
              }
            }
            n202 = Get Date/Time In Seconds() -> (seconds since 1Jan1904=w1033:timestamp)
          }
          frame #3 {
            # "READ POWER OUT"
            n203 = case shown="No Error" w1064 {
              selector: w1064 -> [w1079 w1086]
              tunnel: [w1078 w1086] -> w1072
              tunnel: [w1076 0.0] -> w1067
              tunnel: w1063 -> [w1077 _]
              tunnel: w1062 -> [w1075 w1084]
              tunnel: [w1073 w1084] -> w1069
              frame No Error {
                n204 = call "QUERY POWER OUT M9613.vi"("Communications Port"=w1077, "error in"=w1079) -> ("CRC ERROR"=w1074:bool, "POWER OUT, %"=w1076:dbl, "error out"=w1078:errorcluster)
                n205 = case shown="True" w1074 {
                  selector: w1074 -> [_ w1082]
                  tunnel: w1075 -> [w1080 w1083]
                  tunnel: [w1080 w1081] -> w1073
                  frame False {
                  }
                  frame True {
                    n206 = Bundle By Name(cluster=w1083, "CRC Error"=w1082) -> (w1081:T5)
                  }
                }
              }
              frame Error {
              }
            }
            n207 = case shown="No Error" w1072 {
              selector: w1072 -> [w1089 w1090]
              tunnel: [w1089 w1090] -> w1071
              tunnel: w1067 -> [w1087 _]
              frame No Error {
                n208 = Absolute Value(x=w1087) -> (abs(x)=w1088:dbl)
                n209 = property on="Power" class="Slide (strict)"("Value"=w1088) -> ()  [unwired: 2 in, 2 out]
              }
              frame Error {
              }
            }
            n210 = Build Array (concatenate)(w1066, w1067) -> (w1065:dbl[])
            "Sampling" <- FALSE
          }
          frame #4 {
            n211 = Not Equal To 0?(x=w1099) -> (x != 0?=w1096:bool)
            n212 = And(x="Save Data to File", y=w1096) -> (x .and. y?=w1098:bool)
            n213 = case shown="False" w1098 {
              tunnel: w1097 -> [w1106 w1107]
              tunnel: [w1106 w1107] -> w1094
              frame False {
                "Start Sample Time" <- w1106
              }
              frame True {
              }
            }
            "Sample in Time" <- w1094
            n214 = property on="Start Sample Time" class="AbsTime (strict)"() -> ("Value"=w1104:timestamp)  [unwired: 2 in, 2 out]
            n215 = Subtract(x=w1094, y=w1104) -> (x-y=w1100:dbl)
            "Elapsed Time" <- w1100
            n216 = Build Array (concatenate)(w1100, w1093) -> (w1092:dbl[])
            n217 = case shown="True" "Save Data to File" {
              tunnel: w1105 -> [w1122 w1128]
              tunnel: [w1122 w1124] -> w1102
              tunnel: "Save File" -> [_ w1126]
              tunnel: w1092 -> [_ w1123]
              frame False {
              }
              frame True {
                n218 = Get File Size(file=w1126, error in=w1128) -> (size (in bytes)=w1129:i64, 0:w1127:errorcluster)  [unwired: 1 out]
                n219 = Not Equal To 0?(x=w1129) -> (x != 0?=w1125:bool)
                n220 = case shown="No Error" w1127 {
                  selector: w1127 -> [w1136 w1146]
                  tunnel: w1125 -> [w1138 _]
                  tunnel: w1126 -> [w1137 _]
                  tunnel: w1123 -> [w1134 _]
                  tunnel: [w1130 w1146] -> w1124
                  frame No Error {
                    n221 = case shown="False" w1138 {
                      tunnel: w1137 -> [w1141 w1145]
                      tunnel: [w1141 w1145] -> w1135
                      tunnel: w1136 -> [w1142 w1144]
                      tunnel: [w1143 w1144] -> w1132
                      frame False {
                        n222 = call-poly <vilib>:"Write Delimited Spreadsheet.vi"("file path (dialog if empty)"=w1141, "2D data"=string[][] [["Time", "T_1", "T_2", "T_Set", "Power"], ["[s]", "[C]", "[C]", "[C]", "[%]"]], "error in (no error)"=w1142, "delimiter (\\t)"="," ("delimiter (\\t)")) -> ("error out"=w1143:errorcluster)  [unwired: 10 in, 1 out]
                      }
                      frame True {
                      }
                    }
                    n223 = call-poly <vilib>:"Write Delimited Spreadsheet.vi"("file path (dialog if empty)"=w1135, "1D data"=w1134, "append to file? (new file:F)"=TRUE, "error in (no error)"=w1132, "delimiter (\\t)"="," ("delimiter (\\t)")) -> ("error out"=w1130:errorcluster)  [unwired: 9 in, 1 out]
                  }
                  frame Error {
                  }
                }
              }
            }
            n224 = case shown="Error" w1102 {
              tunnel: w1091 -> [w1108 w1111]
              tunnel: [w1108 w1110] -> w1103
              frame No Error {
              }
              frame Error {
                n225 = Two Button Dialog(message=" Unable to communicate with controller (Error 4), check:\n• Controller is ON and correctly wired\n• Correct communications port is selected\n• Another program is not using the communications port ", 1:"EXIT" ("F button name (\"Cancel\")"), 2:"RESTART" ("T button name (\"OK\")")) -> (T button?=w1109:bool)
                n226 = case shown="True" w1109 {
                  selector: w1109 -> [w1117 _]
                  tunnel: w1111 -> [w1115 w1119]
                  tunnel: [w1116 w1121] -> w1110
                  frame False {
                    n227 = Not(x=w1117) -> (.not. x?=w1118:bool)
                    n228 = Bundle By Name(cluster=w1115, "End"=w1118) -> (w1116:T5)
                  }
                  frame True {
                    w1120 = TRUE
                    n229 = Bundle By Name(cluster=w1119, "Read Model"=w1120, "Read Settings"=w1120) -> (w1121:T5)
                  }
                }
              }
            }
          }
        }
      }
      frame Error {
      }
    }
    n230 = case shown="No Error" w86 {
      selector: w86 -> [w163 w890]
      tunnel: w85 -> [w165 _]
      tunnel: [w164 w890] -> w84
      tunnel: [w162 FALSE] -> w72
      tunnel: w87 -> [w153 w891]
      tunnel: [w153 w891] -> w71
      tunnel: [w161 FALSE ("End")] -> w66
      frame No Error {
        n231 = Multiply(x=i16 1000, y="Sample Rate (s)") -> (x*y=w154:i16)
        n232 = In Range and Coerce(upper limit=inf, x=w154, lower limit=i16 0) -> (coerced(x)=w159:dbl)  [unwired: 1 out]
        n233 = event shown="[15] \"Control Settings.Proportional Bandwidth\": Value Change" {
          selector: _ -> [_ _ _ _ _ _ _ _ _ _ _ _ _ _ _ _ _ _ _ _ _ _ _ _]
          dyn-events: _ -> [_ _ _ _ _ _ _ _ _ _ _ _ _ _ _ _ _ _ _ _ _ _ _ _]
          timeout: w159 -> [_ _ _ _ _ _ _ _ _ _ _ _ _ _ _ _ _ _ _ _ _ _ _ _]
          tunnel: [w171 w184 w205 w223 w240 w262 w296 w335 w375 w409 w448 w491 w509 w524 w578 w630 w673 w720 w767 w782 w803 w826 w859 w887] -> w164
          tunnel: [w170 w185 w204 w222 w241 w261 w299 w336 w374 w404 w451 w488 w506 w523 w577 w628 w677 w723 w766 w781 w805 w827 w857 w886] -> w162
          tunnel: FALSE -> [w169 _ w202 w220 w239 w267 w304 w341 w379 w417 w457 w490 w508 w526 w580 w627 w678 w724 w765 w783 w804 w825 w861 w886]
          tunnel: w163 -> [w168 w187 w201 w219 w238 w266 w303 w342 w380 w416 w456 w489 w507 w525 w579 w631 w676 w719 w768 w784 w806 w830 w856 w887]
          tunnel: w165 -> [w167 w188 w200 w218 w237 w265 w302 w340 w378 w415 w455 w487 w505 w527 w581 w632 w675 w722 w764 w785 w802 w831 w863 _]
          tunnel: [w166 w183 w199 w217 w235 w258 w293 w332 w370 w407 w444 w486 w503 w521 w575 w625 w670 w716 w763 w780 w800 w819 w854 _] -> w161
          event "Output Polarity": Value Change {
            n234 = event-data() -> ("NewVal"=w172:enum32{"Cool", "Heat "})  [unwired: 1 in]
            n235 = case shown="No Error" w168 {
              selector: w168 -> [w177 w182]
              tunnel: w172 -> [w179 _]
              tunnel: [w178 w182] -> w171
              tunnel: [w176 w181] -> w170
              tunnel: w169 -> [_ w181]
              tunnel: w167 -> [w175 _]
              tunnel: [w173 FALSE ("End")] -> w166
              frame No Error {
                n236 = call "SEND COMMAND TC-48-20.vi"("Communications Port"=w175, "Format String"="21%04x", "error in"=w177, "Data"=w179) -> ("CRC ERROR"=w176:bool, "End"=w173:bool, "error out"=w178:errorcluster)  [unwired: 1 in]
              }
              frame Error {
              }
            }
          }
          event "Alarm Latch": Value Change {
            n237 = event-data() -> ("NewVal"=w186:T2)  [unwired: 1 in]
            n238 = case shown="No Error" w187 {
              selector: w187 -> [w194 w198]
              tunnel: [w195 FALSE] -> w185
              tunnel: [w193 w198] -> w184
              tunnel: w188 -> [w192 _]
              tunnel: w186 -> [w191 _]
              tunnel: [w189 FALSE ("End")] -> w183
              frame No Error {
                n239 = call "SEND COMMAND TC-48-20.vi"("Communications Port"=w192, "Format String"="2b%04x", "error in"=w194, "Data"=w191) -> ("CRC ERROR"=w195:bool, "End"=w189:bool, "error out"=w193:errorcluster)  [unwired: 1 in]
              }
              frame Error {
              }
            }
          }
          event "Shutdown Output w/ Alarm 2": Value Change {
            n240 = event-data() -> ("NewVal"=w203:bool)  [unwired: 1 in]
            n241 = case shown="No Error" w201 {
              selector: w201 -> [w211 w216]
              tunnel: [w213 w215] -> w204
              tunnel: [w212 w216] -> w205
              tunnel: w203 -> [w210 _]
              tunnel: w202 -> [_ w215]
              tunnel: w200 -> [w209 _]
              tunnel: [w206 FALSE ("End")] -> w199
              frame No Error {
                n242 = Boolean To (0,1)(Boolean=w210) -> (0, 1=w207:i16)
                n243 = call "SEND COMMAND TC-48-20.vi"("Communications Port"=w209, "Format String"="2a%04x", "error in"=w211, "Data"=w207) -> ("CRC ERROR"=w213:bool, "End"=w206:bool, "error out"=w212:errorcluster)  [unwired: 1 in]
              }
              frame Error {
              }
            }
          }
          event "Shutdown Output w/ Alarm 1": Value Change {
            n244 = event-data() -> ("NewVal"=w221:bool)  [unwired: 1 in]
            n245 = case shown="No Error" w219 {
              selector: w219 -> [w229 w234]
              tunnel: [w231 w233] -> w222
              tunnel: [w230 w234] -> w223
              tunnel: w221 -> [w228 _]
              tunnel: w220 -> [_ w233]
              tunnel: w218 -> [w227 _]
              tunnel: [w224 FALSE ("End")] -> w217
              frame No Error {
                n246 = Boolean To (0,1)(Boolean=w228) -> (0, 1=w225:i16)
                n247 = call "SEND COMMAND TC-48-20.vi"("Communications Port"=w227, "Format String"="27%04x", "error in"=w229, "Data"=w225) -> ("CRC ERROR"=w231:bool, "End"=w224:bool, "error out"=w230:errorcluster)  [unwired: 1 in]
              }
              frame Error {
              }
            }
          }
          event "Clear Alarm Latch": Value Change {
            n248 = event-data() -> ("OldVal"=w236:bool)  [unwired: 1 in]
            n249 = case shown="No Error" w238 {
              selector: w238 -> [w248 w252]
              tunnel: [w249 w252] -> w240
              tunnel: [w247 w251] -> w241
              tunnel: w239 -> [_ w251]
              tunnel: w237 -> [w246 _]
              tunnel: w236 -> [w244 _]
              tunnel: [w242 FALSE ("End")] -> w235
              frame No Error {
                n250 = Boolean To (0,1)(Boolean=w244) -> (0, 1=w243:i16)
                n251 = call "SEND COMMAND TC-48-20.vi"("Communications Port"=w246, "Format String"="33%04x", "error in"=w248, "Data"=w243) -> ("CRC ERROR"=w247:bool, "End"=w242:bool, "error out"=w249:errorcluster)  [unwired: 1 in]
              }
              frame Error {
              }
            }
          }
          event "Alarm 1 High": Value Change {
            n252 = event-data() -> ("NewVal"=w254:dbl, "OldVal"=w257:dbl)  [unwired: 1 in]
            n253 = In Range and Coerce(upper limit=200.0, x=w254, lower limit=-inf) -> (coerced(x)=w253:dbl)  [unwired: 1 out]
            n254 = case shown="No Error" w266 {
              selector: w266 -> [w281 w287]
              tunnel: w253 -> [w277 _]
              tunnel: [w282 w287] -> w264
              tunnel: [w280 w286] -> w260
              tunnel: w267 -> [_ w286]
              tunnel: w265 -> [w278 w284]
              tunnel: [w277 inf] -> _
              tunnel: [w278 w284] -> w263
              tunnel: [w276 FALSE ("End")] -> w258
              frame No Error {
                n255 = call "SEND COMMAND TC-48-20.vi"("Communications Port"=w278, "Format String"="26%04x", "error in"=w281, "Data"=w277) -> ("CRC ERROR"=w280:bool, "End"=w276:bool, "error out"=w282:errorcluster)  [unwired: 1 in]
              }
              frame Error {
              }
            }
            n256 = case shown="No Error" w264 {
              selector: w264 -> [w271 w275]
              tunnel: w263 -> [w272 _]
              tunnel: [w270 w275] -> w262
              tunnel: [w269 w274] -> w261
              tunnel: w260 -> [_ w274]
              tunnel: [w268 w273] -> w259
              tunnel: w257 -> [_ w273]
              frame No Error {
                n257 = call "QUERY HIGH ALARM SET POINT M9613.vi"("Communications Port"=w272, "error in"=w271) -> ("CRC ERROR"=w269:bool, "HIGH ALARM SETPOINT INPUT 1"=w268:dbl, "error out"=w270:errorcluster)
              }
              frame Error {
              }
            }
            n258 = property on="Alarm 1 High" class="DigNum (strict)"("Value"=w259) -> ()  [unwired: 2 in, 2 out]
          }
          event "Alarm 2 High": Value Change {
            n259 = event-data() -> ("NewVal"=w290:dbl, "OldVal"=w292:dbl)  [unwired: 1 in]
            n260 = In Range and Coerce(upper limit=200.0, x=w290, lower limit=-inf) -> (coerced(x)=w289:dbl)  [unwired: 1 out]
            n261 = case shown="No Error" w303 {
              selector: w303 -> [w320 w325]
              tunnel: w289 -> [w316 _]
              tunnel: [w321 w325] -> w301
              tunnel: [w319 w324] -> w300
              tunnel: w304 -> [_ w324]
              tunnel: w302 -> [w317 w323]
              tunnel: [w317 w323] -> w297
              tunnel: [w315 FALSE ("End")] -> w295
              frame No Error {
                n262 = call "SEND COMMAND TC-48-20.vi"("Communications Port"=w317, "Format String"="29%04x", "error in"=w320, "Data"=w316) -> ("CRC ERROR"=w319:bool, "End"=w315:bool, "error out"=w321:errorcluster)  [unwired: 1 in]
              }
              frame Error {
              }
            }
            n263 = case shown="No Error" w301 {
              selector: w301 -> [w310 w314]
              tunnel: [w309 w314] -> w296
              tunnel: [w308 w313] -> w299
              tunnel: [w307 w312] -> w298
              tunnel: w300 -> [_ w313]
              tunnel: w292 -> [_ w312]
              tunnel: w297 -> [w306 _]
              tunnel: [w305 FALSE ("End")] -> w294
              frame No Error {
                n264 = call "QUERY HIGH ALARM SET POINT INPUT 2 M9613.vi"("Communications Port"=w306, "error in"=w310) -> ("CRC ERROR"=w308:bool, "End"=w305:bool, "HIGH ALARM SETPOINT INPUT 2"=w307:dbl, "error out"=w309:errorcluster)
              }
              frame Error {
              }
            }
            n265 = property on="Alarm 2 High" class="DigNum (strict)"("Value"=w298) -> ()  [unwired: 2 in, 2 out]
            n266 = Or(x=w295, y=w294) -> (x .or. y?=w293:bool)
          }
          event "Alarm 1 Low": Value Change {
            n267 = event-data() -> ("NewVal"=w327:dbl, "OldVal"=w330:dbl)  [unwired: 1 in]
            n268 = In Range and Coerce(upper limit=inf, x=w327, lower limit=-21.0) -> (coerced(x)=w326:dbl)  [unwired: 1 out]
            n269 = case shown="No Error" w342 {
              selector: w342 -> [w358 w363]
              tunnel: w326 -> [w354 _]
              tunnel: [w359 w363] -> w339
              tunnel: [w357 w362] -> w337
              tunnel: w341 -> [_ w362]
              tunnel: w340 -> [w355 w361]
              tunnel: [w355 w361] -> w334
              tunnel: [w353 FALSE ("End")] -> w333
              frame No Error {
                n270 = call "SEND COMMAND TC-48-20.vi"("Communications Port"=w355, "Format String"="25%04x", "error in"=w358, "Data"=w354) -> ("CRC ERROR"=w357:bool, "End"=w353:bool, "error out"=w359:errorcluster)  [unwired: 1 in]
              }
              frame Error {
              }
            }
            n271 = case shown="No Error" w339 {
              selector: w339 -> [w348 w352]
              tunnel: [w347 w352] -> w335
              tunnel: [w346 w350] -> w336
              tunnel: [w345 w351] -> w338
              tunnel: w330 -> [_ w351]
              tunnel: w337 -> [_ w350]
              tunnel: w334 -> [w344 _]
              tunnel: [w343 FALSE ("End")] -> w331
              frame No Error {
                n272 = call "QUERY LOW ALARM SET POINT M9613.vi"("Communications Port"=w344, "error in"=w348) -> ("CRC ERROR"=w346:bool, "End"=w343:bool, "LOW ALARM SETPOINT"=w345:dbl, "error out"=w347:errorcluster)
              }
              frame Error {
              }
            }
            n273 = property on="Alarm 2 Low" class="DigNum (strict)"("Value"=w338) -> ()  [unwired: 2 in, 2 out]
            n274 = Or(x=w333, y=w331) -> (x .or. y?=w332:bool)
          }
          event "Alarm 2 Low": Value Change {
            n275 = event-data() -> ("NewVal"=w365:dbl, "OldVal"=w368:dbl)  [unwired: 1 in]
            n276 = In Range and Coerce(upper limit=inf, x=w365, lower limit=-21.0) -> (coerced(x)=w364:dbl)  [unwired: 1 out]
            n277 = case shown="No Error" w380 {
              selector: w380 -> [w397 w403]
              tunnel: w364 -> [w399 _]
              tunnel: [w398 w403] -> w377
              tunnel: [w396 w402] -> w376
              tunnel: w379 -> [_ w402]
              tunnel: w378 -> [w392 w401]
              tunnel: [w392 w401] -> w373
              tunnel: [w391 FALSE ("End")] -> w371
              frame No Error {
                n278 = Multiply(x=1, y=w399) -> (x*y=w394:dbl)
                n279 = call "SEND COMMAND TC-48-20.vi"("Communications Port"=w392, "Format String"="28%04x", "error in"=w397, "Data"=w394) -> ("CRC ERROR"=w396:bool, "End"=w391:bool, "error out"=w398:errorcluster)  [unwired: 1 in]
              }
              frame Error {
              }
            }
            n280 = case shown="Error" w377 {
              selector: w377 -> [w386 w390]
              tunnel: [w385 w390] -> w375
              tunnel: [w384 w389] -> w374
              tunnel: [w383 w388] -> w372
              tunnel: w376 -> [_ w389]
              tunnel: w368 -> [_ w388]
              tunnel: w373 -> [w382 _]
              tunnel: [w381 FALSE ("End")] -> w369
              frame No Error {
                n281 = call "QUERY LOW ALARM SET POINT INPUT 2 M9613.vi"("Communications Port"=w382, "error in"=w386) -> ("CRC ERROR"=w384:bool, "End"=w381:bool, "LOW ALARM SETPOINT INPUT 2"=w383:dbl, "error out"=w385:errorcluster)
              }
              frame Error {
              }
            }
            n282 = property on="Alarm 2 Low" class="DigNum (strict)"("Value"=w372) -> ()  [unwired: 2 in, 2 out]
            n283 = Or(x=w371, y=w369) -> (x .or. y?=w370:bool)
          }
          event "Alarm 1 Deadband": Value Change {
            n284 = event-data() -> ("NewVal"=w418:dbl)  [unwired: 1 in]
            n285 = Multiply(x=w418, y=10) -> (x*y=w410:dbl)
            n286 = case shown="No Error" w416 {
              selector: w416 -> [w437 w443]
              tunnel: w410 -> [w439 _]
              tunnel: [w438 w443] -> w413
              tunnel: [w436 w442] -> w412
              tunnel: w417 -> [_ w442]
              tunnel: w415 -> [w434 w441]
              tunnel: [w434 w441] -> w411
              tunnel: [w433 FALSE ("End")] -> w408
              frame No Error {
                n287 = call "SEND COMMAND TC-48-20.vi"("Communications Port"=w434, "Format String"="2d%04x", "error in"=w437, "Data"=w439) -> ("CRC ERROR"=w436:bool, "End"=w433:bool, "error out"=w438:errorcluster)  [unwired: 1 in]
              }
              frame Error {
              }
            }
            n288 = case shown="No Error" w413 {
              selector: w413 -> [w430 w432]
              tunnel: w411 -> [w429 _]
              tunnel: [w427 w432] -> w409
              tunnel: w410 -> [w421 _]
              tunnel: [w426 w431] -> w406
              tunnel: [w425 w431] -> w405
              frame No Error {
                n289 = call "QUERY ALARM 1 DEADBAND M9613.vi"("Communications Port"=w429, "error in"=w430) -> ("CRC ERROR"=w425:bool, "End"=w426:bool, "ALARM 1 DEADBAND"=w420:dbl, "error out"=w428:errorcluster)
                n290 = Subtract(x=w420, y=w421) -> (x-y=w424:dbl)
                n291 = Absolute Value(x=w424) -> (abs(x)=w423:dbl)
                n292 = Greater?(x=w423, y=0.01) -> (0:w419:bool)
                n293 = Bundle By Name(cluster=w428, "status"=w419) -> (w427:errorcluster)
              }
              frame Error {
                w431 = FALSE ("End")
              }
            }
            n294 = Or(x=w412, y=w405) -> (x .or. y?=w404:bool)
            n295 = Or(x=w408, y=w406) -> (x .or. y?=w407:bool)
          }
          event "Alarm 2 Deadband": Value Change {
            n296 = event-data() -> ("NewVal"=w458:dbl)  [unwired: 1 in]
            n297 = Multiply(x=w458, y=10) -> (x*y=w454:dbl)
            n298 = case shown="No Error" w456 {
              selector: w456 -> [w479 w485]
              tunnel: w454 -> [w475 w482]
              tunnel: [w480 w485] -> w452
              tunnel: [w478 w484] -> w450
              tunnel: w457 -> [_ w484]
              tunnel: w455 -> [w476 w483]
              tunnel: [w476 w483] -> w449
              tunnel: [w475 w482] -> w447
              tunnel: [w474 FALSE ("End")] -> w446
              frame No Error {
                n299 = call "SEND COMMAND TC-48-20.vi"("Communications Port"=w476, "Format String"="2e%04x", "error in"=w479, "Data"=w475) -> ("CRC ERROR"=w478:bool, "End"=w474:bool, "error out"=w480:errorcluster)  [unwired: 1 in]
              }
              frame Error {
              }
            }
            n300 = case shown="No Error" w452 {
              selector: w452 -> [w470 w472]
              tunnel: [w469 w473] -> w451
              tunnel: w450 -> [_ w473]
              tunnel: w449 -> [w468 _]
              tunnel: [w466 w472] -> w448
              tunnel: w447 -> [w461 _]
              tunnel: [w465 FALSE ("END")] -> w445
              frame No Error {
                n301 = call "QUERY ALARM 2 DEADBAND M9613.vi"("error in"=w470, "Communications Port"=w468) -> ("error out"=w467:errorcluster, "ALARM 2 DEADBAND"=w460:dbl, "END"=w465:bool, "CRC ERROR"=w469:bool)  [unwired: 1 in]
                n302 = Subtract(x=w460, y=w461) -> (x-y=w464:dbl)
                n303 = Absolute Value(x=w464) -> (abs(x)=w463:dbl)
                n304 = Greater?(x=w463, y=0.01) -> (0:w459:bool)
                n305 = Bundle By Name(cluster=w467, "status"=w459) -> (w466:errorcluster)
              }
              frame Error {
              }
            }
            n306 = Or(x=w446, y=w445) -> (x .or. y?=w444:bool)
          }
          event "Sensor Type": Value Change {
            n307 = event-data() -> ("NewVal"=w492:enum32{"15K", "10K"})  [unwired: 1 in, 5 out]
            n308 = case shown="No Error" w489 {
              selector: w489 -> [w496 w502]
              tunnel: [w498 w502] -> w491
              tunnel: [w497 w501] -> w488
              tunnel: w492 -> [w495 _]
              tunnel: w490 -> [_ w501]
              tunnel: w487 -> [w494 _]
              tunnel: [w493 FALSE ("End")] -> w486
              frame No Error {
                n309 = call "SEND COMMAND TC-48-20.vi"("Communications Port"=w494, "Format String"="20%04x", "error in"=w496, "Data"=w495) -> ("CRC ERROR"=w497:bool, "End"=w493:bool, "error out"=w498:errorcluster)  [unwired: 1 in]
              }
              frame Error {
              }
            }
          }
          event "Run Peltier": Value Change {
            n310 = event-data() -> ("NewVal"=w510:bool)  [unwired: 1 in]
            n311 = Boolean To (0,1)(Boolean=w510) -> (0, 1=w504:i16)
            n312 = case shown="No Error" w507 {
              selector: w507 -> [w514 w520]
              tunnel: [w516 w520] -> w509
              tunnel: [w515 w519] -> w506
              tunnel: w504 -> [w513 _]
              tunnel: w508 -> [_ w519]
              tunnel: w505 -> [w512 _]
              tunnel: [w511 FALSE ("End")] -> w503
              frame No Error {
                n313 = call "SEND COMMAND TC-48-20.vi"("Communications Port"=w512, "Format String"="30%04x", "error in"=w514, "Data"=w513) -> ("CRC ERROR"=w515:bool, "End"=w511:bool, "error out"=w516:errorcluster)  [unwired: 1 in]
              }
              frame Error {
              }
            }
          }
          event "Set Temperature": Value Change {
            n314 = event-data() -> ("NewVal"=w522:dbl)  [unwired: 1 in]
            n315 = case shown="No Error" w525 {
              selector: w525 -> [w544 w574]
              tunnel: w526 -> [w535 w573]
              tunnel: w527 -> [w541 _]
              tunnel: w522 -> [w528 _]
              tunnel: [w542 w574] -> w524
              tunnel: [w536 w573] -> w523
              tunnel: [w534 FALSE ("End")] -> w521
              frame No Error {
                n316 = property on="Set Limit High" class="DigNum (strict)"() -> ("Value"=w531:dbl)  [unwired: 2 in, 2 out]
                n317 = property on="Set Limit Low" class="DigNum (strict)"() -> ("Value"=w530:dbl)  [unwired: 2 in, 2 out]
                n318 = In Range and Coerce(upper limit=w531, x=w528, lower limit=w530) -> (coerced(x)=w529:dbl)  [unwired: 1 out]
                n319 = Multiply(x=10, y=w529) -> (x*y=w540:dbl)
                n320 = case shown="No Error" w544 {
                  selector: w544 -> [w567 w571]
                  tunnel: [w568 w571] -> w543
                  tunnel: [w566 w570] -> w538
                  tunnel: w535 -> [_ w570]
                  tunnel: w541 -> [w565 _]
                  tunnel: w540 -> [w563 _]
                  tunnel: [w562 FALSE ("End")] -> w532
                  frame No Error {
                    n321 = call "SEND COMMAND TC-48-20.vi"("Communications Port"=w565, "Format String"="1c%04x", "error in"=w567, "Data"=w563) -> ("CRC ERROR"=w566:bool, "End"=w562:bool, "error out"=w568:errorcluster)  [unwired: 1 in]
                  }
                  frame Error {
                  }
                }
                n322 = case shown="No Error" w543 {
                  selector: w543 -> [w552 w561]
                  tunnel: [w555 w559] -> w542
                  tunnel: [w556 TRUE] -> w537
                  tunnel: w541 -> [w553 _]
                  tunnel: w529 -> [w547 _]
                  tunnel: [w545 FALSE ("End")] -> w533
                  frame No Error {
                    n323 = call "QUERY SETPOINT M9613.vi"("Communications Port"=w553, "error in"=w552) -> ("CRC ERROR"=w556:bool, "End"=w545:bool, "SET POINT"=w546:dbl, "error out"=w554:errorcluster)
                    n324 = Subtract(x=w546, y=w547) -> (x-y=w551:dbl)
                    n325 = Absolute Value(x=w551) -> (abs(x)=w550:dbl)
                    n326 = Greater?(x=w550, y=0.01) -> (0:w548:bool)
                    n327 = Bundle By Name(cluster=w554, "status"=w548) -> (w555:errorcluster)
                  }
                  frame Error {
                    n328 = call <vilib>:"Simple Error Handler.vi"("error source (\" \")"="SET TEMPERATURE ERROR", "error in (no error)"=w561) -> ("error out"=w559:errorcluster)  [unwired: 3 in, 4 out]
                  }
                }
                n329 = Or(x=w532, y=w533) -> (x .or. y?=w534:bool)
                n330 = Compound Arithmetic op=OR(w538, w537) -> (w536:bool)
              }
              frame Error {
              }
            }
          }
          event "Temperature 2 Display": Value Change {
            n331 = event-data() -> ("NewVal"=w576:T3)  [unwired: 1 in]
            n332 = case shown="No Error" w579 {
              selector: w579 -> [w592 w623]
              tunnel: w580 -> [w593 w622]
              tunnel: w581 -> [w589 _]
              tunnel: w576 -> [w585 _]
              tunnel: [w590 w623] -> w578
              tunnel: [w586 w622] -> w577
              tunnel: [w582 FALSE ("End")] -> w575
              frame No Error {
                n333 = case shown="No Error" w592 {
                  selector: w592 -> [w616 w620]
                  tunnel: [w617 w620] -> w591
                  tunnel: [w615 w619] -> w588
                  tunnel: w593 -> [_ w619]
                  tunnel: w589 -> [w614 _]
                  tunnel: [w612 FALSE ("End")] -> w583
                  tunnel: w585 -> [w611 _]
                  frame No Error {
                    n334 = call "SEND COMMAND TC-48-20.vi"("Communications Port"=w614, "Format String"="2c%04x", "error in"=w616, "Data"=w611) -> ("CRC ERROR"=w615:bool, "End"=w612:bool, "error out"=w617:errorcluster)  [unwired: 1 in]
                  }
                  frame Error {
                  }
                }
                n335 = case shown="No Error" w591 {
                  selector: w591 -> [w601 w610]
                  tunnel: [w604 w608] -> w590
                  tunnel: [w605 TRUE] -> w587
                  tunnel: w589 -> [w602 _]
                  tunnel: w585 -> [w595 _]
                  tunnel: [w600 FALSE ("End")] -> w584
                  frame No Error {
                    n336 = call "QUERY TEMP 2 DISPLAY M9613.vi"("Communications Port"=w602, "error in"=w601) -> ("CRC ERROR"=w605:bool, "End"=w600:bool, "TEMPERATURE 2 DISPLAY"=w596:dbl, "error out"=w603:errorcluster)
                    n337 = Subtract(x=w595, y=w596) -> (x-y=w599:dbl)
                    n338 = Absolute Value(x=w599) -> (abs(x)=w598:dbl)
                    n339 = Greater?(x=w598, y=0.01) -> (0:w594:bool)
                    n340 = Bundle By Name(cluster=w603, "status"=w594) -> (w604:errorcluster)
                  }
                  frame Error {
                    n341 = call <vilib>:"Simple Error Handler.vi"("error source (\" \")"="SET TEMPERATURE ERROR", "error in (no error)"=w610) -> ("error out"=w608:errorcluster)  [unwired: 3 in, 4 out]
                  }
                }
                n342 = Or(x=w583, y=w584) -> (x .or. y?=w582:bool)
                n343 = Or(x=w588, y=w587) -> (x .or. y?=w586:bool)
              }
              frame Error {
              }
            }
          }
          event "Control Settings.Proportional Bandwidth": Value Change {
            n344 = event-data() -> ("NewVal"=w629:dbl)  [unwired: 1 in]
            n345 = case shown="No Error" w631 {
              selector: w631 -> [w638 w669]
              tunnel: [w640 w665] -> w628
              tunnel: [w641 w668] -> w630
              tunnel: w632 -> [w635 _]
              tunnel: w629 -> [w636 _]
              tunnel: w627 -> [_ w665]
              tunnel: [w634 w664] -> w626
              tunnel: [w633 w664] -> w624
              frame No Error {
                n346 = case shown="No Error" w638 {
                  selector: w638 -> [w658 w663]
                  tunnel: [w660 w663] -> w637
                  tunnel: [w657 TRUE] -> w642
                  tunnel: w635 -> [w656 _]
                  tunnel: w636 -> [w654 _]
                  tunnel: [w652 FALSE ("End")] -> w634
                  frame No Error {
                    n347 = Multiply(x=w654, y=10) -> (x*y=w653:dbl)
                    n348 = call "SEND COMMAND TC-48-20.vi"("Communications Port"=w656, "Format String"="1d%04x", "error in"=w658, "Data"=w653) -> ("CRC ERROR"=w657:bool, "End"=w652:bool, "error out"=w660:errorcluster)  [unwired: 1 in]
                  }
                  frame Error {
                  }
                }
                n349 = case shown="No Error" w637 {
                  selector: w637 -> [w646 w651]
                  tunnel: [w645 w651] -> w641
                  tunnel: [w648 TRUE] -> w639
                  tunnel: w635 -> [w647 _]
                  tunnel: [w643 FALSE ("End")] -> w633
                  frame No Error {
                    n350 = call "QUERY PROPORTIONAL BW M9613.vi"("Communications Port"=w647, "error in"=w646) -> ("CRC ERROR"=w648:bool, "End"=w643:bool, "PROPOTIONAL BW"=w644:dbl, "error out"=w645:errorcluster)
                    n351 = property on="Proportional Bandwidth" class="DigNum (strict)"("Value"=w644) -> ()  [unwired: 2 in, 2 out]
                  }
                  frame Error {
                  }
                }
                n352 = Or(x=w642, y=w639) -> (x .or. y?=w640:bool)
              }
              frame Error {
                w664 = FALSE ("End")
                w666 = T9 2 items=["no dialog", "OK message", "continue or stop message", "OK message + warnings", "continue/stop + warnings"] ("type of dialog (OK msg:1)")
                n353 = call <vilib>:"Simple Error Handler.vi"("error source (\" \")"="PROPORTIONAL SEND ERROR", "type of dialog (OK msg:1)"=w666, "error in (no error)"=w669) -> ("error out"=w668:errorcluster)  [unwired: 2 in, 4 out]
              }
            }
            n354 = Or(x=w626, y=w624) -> (x .or. y?=w625:bool)
          }
          event "Control Settings.Integral Gain": Value Change {
            n355 = event-data() -> ("NewVal"=w674:dbl)  [unwired: 1 in]
            n356 = case shown="No Error" w676 {
              selector: w676 -> [w684 w715]
              tunnel: [w686 w711] -> w677
              tunnel: [w687 w714] -> w673
              tunnel: w675 -> [w681 _]
              tunnel: w674 -> [w682 _]
              tunnel: w678 -> [_ w711]
              tunnel: [w680 w710] -> w671
              tunnel: [w679 w710] -> w672
              frame No Error {
                n357 = case shown="No Error" w684 {
                  selector: w684 -> [w704 w709]
                  tunnel: [w706 w709] -> w683
                  tunnel: [w703 TRUE] -> w688
                  tunnel: w681 -> [w702 _]
                  tunnel: w682 -> [w700 _]
                  tunnel: [w698 FALSE ("End")] -> w680
                  frame No Error {
                    n358 = Multiply(x=w700, y=100) -> (x*y=w701:dbl)
                    n359 = call "SEND COMMAND TC-48-20.vi"("Communications Port"=w702, "Format String"="1e%04x", "error in"=w704, "Data"=w701) -> ("CRC ERROR"=w703:bool, "End"=w698:bool, "error out"=w706:errorcluster)  [unwired: 1 in]
                  }
                  frame Error {
                  }
                }
                n360 = case shown="No Error" w683 {
                  selector: w683 -> [w692 w697]
                  tunnel: [w691 w697] -> w687
                  tunnel: [w694 TRUE] -> w685
                  tunnel: w681 -> [w693 _]
                  tunnel: [w689 FALSE ("End")] -> w679
                  frame No Error {
                    n361 = call "QUERY INTEGRAL GAIN M9613.vi"("Communications Port"=w693, "error in"=w692) -> ("CRC ERROR"=w694:bool, "End"=w689:bool, "INTEGRAL GAIN"=w690:dbl, "error out"=w691:errorcluster)
                    n362 = property on="Integral Gain" class="DigNum (strict)"("Value"=w690) -> ()  [unwired: 2 in, 2 out]
                  }
                  frame Error {
                  }
                }
                n363 = Or(x=w688, y=w685) -> (x .or. y?=w686:bool)
              }
              frame Error {
                w710 = FALSE ("End")
                w712 = T9 2 items=["no dialog", "OK message", "continue or stop message", "OK message + warnings", "continue/stop + warnings"] ("type of dialog (OK msg:1)")
                n364 = call <vilib>:"Simple Error Handler.vi"("error source (\" \")"="INTEGRAL ERROR", "type of dialog (OK msg:1)"=w712, "error in (no error)"=w715) -> ("error out"=w714:errorcluster)  [unwired: 2 in, 4 out]
              }
            }
            n365 = Or(x=w671, y=w672) -> (x .or. y?=w670:bool)
          }
          event "Control Settings.Derivative Gain": Value Change {
            n366 = event-data() -> ("NewVal"=w721:dbl)  [unwired: 1 in]
            n367 = case shown="No Error" w719 {
              selector: w719 -> [w730 w761]
              tunnel: [w732 w757] -> w723
              tunnel: [w733 w760] -> w720
              tunnel: w722 -> [w727 _]
              tunnel: w721 -> [w728 _]
              tunnel: w724 -> [_ w757]
              tunnel: [w726 w756] -> w718
              tunnel: [w725 w756] -> w717
              frame No Error {
                n368 = case shown="No Error" w730 {
                  selector: w730 -> [w750 w755]
                  tunnel: [w752 w755] -> w729
                  tunnel: [w749 TRUE] -> w734
                  tunnel: w727 -> [w748 _]
                  tunnel: w728 -> [w747 _]
                  tunnel: [w744 FALSE ("End")] -> w726
                  frame No Error {
                    n369 = Multiply(x=w747, y=100) -> (x*y=w745:dbl)
                    n370 = call "SEND COMMAND TC-48-20.vi"("Communications Port"=w748, "Format String"="1f%04x", "error in"=w750, "Data"=w745) -> ("CRC ERROR"=w749:bool, "End"=w744:bool, "error out"=w752:errorcluster)  [unwired: 1 in]
                  }
                  frame Error {
                  }
                }
                n371 = case shown="No Error" w729 {
                  selector: w729 -> [w737 w743]
                  tunnel: [w738 w743] -> w733
                  tunnel: [w740 TRUE] -> w731
                  tunnel: w727 -> [w739 _]
                  tunnel: [w735 FALSE ("End")] -> w725
                  frame No Error {
                    n372 = call "QUERY DERIVATIVE GAIN M9613.vi"("Communications Port"=w739, "error in"=w737) -> ("CRC ERROR"=w740:bool, "End"=w735:bool, "DERIVATIVE GAIN"=w736:dbl, "error out"=w738:errorcluster)
                    n373 = property on="Derivative Gain" class="DigNum (strict)"("Value"=w736) -> ()  [unwired: 2 in, 2 out]
                  }
                  frame Error {
                  }
                }
                n374 = Or(x=w734, y=w731) -> (x .or. y?=w732:bool)
              }
              frame Error {
                w756 = FALSE ("End")
                w758 = T9 2 items=["no dialog", "OK message", "continue or stop message", "OK message + warnings", "continue/stop + warnings"] ("type of dialog (OK msg:1)")
                n375 = call <vilib>:"Simple Error Handler.vi"("error source (\" \")"="DERATIVE ERROR", "type of dialog (OK msg:1)"=w758, "error in (no error)"=w761) -> ("error out"=w760:errorcluster)  [unwired: 2 in, 4 out]
              }
            }
            n376 = Or(x=w718, y=w717) -> (x .or. y?=w716:bool)
          }
          event "Control Settings.Set Limit High": Value Change {
            n377 = event-data() -> ("NewVal"=w762:dbl)  [unwired: 1 in]
            n378 = case shown="No Error" w768 {
              selector: w768 -> [w774 w778]
              tunnel: [w775 w778] -> w767
              tunnel: [w773 w777] -> w766
              tunnel: w762 -> [w771 _]
              tunnel: w765 -> [_ w777]
              tunnel: w764 -> [w770 _]
              tunnel: [w769 FALSE ("End")] -> w763
              frame No Error {
                n379 = call "SEND COMMAND TC-48-20.vi"("Communications Port"=w770, "Format String"="23%04x", "error in"=w774, "Data"=w771) -> ("CRC ERROR"=w773:bool, "End"=w769:bool, "error out"=w775:errorcluster)  [unwired: 1 in]
              }
              frame Error {
              }
            }
          }
          event "Control Settings.Set Limit Low": Value Change {
            n380 = event-data() -> ("NewVal"=w779:dbl)  [unwired: 1 in]
            n381 = case shown="No Error" w784 {
              selector: w784 -> [w791 w795]
              tunnel: [w792 w795] -> w782
              tunnel: [w790 w794] -> w781
              tunnel: w783 -> [_ w794]
              tunnel: w785 -> [w789 _]
              tunnel: w779 -> [w787 _]
              tunnel: [w786 FALSE ("End")] -> w780
              frame No Error {
                n382 = call "SEND COMMAND TC-48-20.vi"("Communications Port"=w789, "Format String"="22%04x", "error in"=w791, "Data"=w787) -> ("CRC ERROR"=w790:bool, "End"=w786:bool, "error out"=w792:errorcluster)  [unwired: 1 in]
              }
              frame Error {
              }
            }
          }
          event "Analog Output Multiplier": Value Change {
            n383 = event-data() -> ("NewVal"=w801:dbl)  [unwired: 1 in]
            n384 = Absolute Value(x=w801) -> (abs(x)=w797:dbl)
            n385 = In Range and Coerce(upper limit=100.0, x=w797, lower limit=-inf) -> (coerced(x)=w796:dbl)  [unwired: 1 out]
            n386 = case shown="No Error" w806 {
              selector: w806 -> [w814 w818]
              tunnel: [w815 w818] -> w803
              tunnel: [w813 w817] -> w805
              tunnel: w796 -> [w810 _]
              tunnel: w804 -> [_ w817]
              tunnel: w802 -> [w811 _]
              tunnel: [w807 FALSE ("End")] -> w800
              frame No Error {
                n387 = Multiply(x=w810, y=100) -> (x*y=w808:dbl)
                n388 = call "SEND COMMAND TC-48-20.vi"("Communications Port"=w811, "Format String"="2f%04x", "error in"=w814, "Data"=w808) -> ("CRC ERROR"=w813:bool, "End"=w807:bool, "error out"=w815:errorcluster)  [unwired: 1 in]
              }
              frame Error {
              }
            }
          }
          event "Control Settings.Control Sensor Offset": Value Change {
            n389 = event-data() -> ("NewVal"=w832:dbl)  [unwired: 1 in]
            n390 = Multiply(x=w832, y=10) -> (x*y=w823:dbl)
            n391 = case shown="No Error" w830 {
              selector: w830 -> [w847 w852]
              tunnel: [w848 w852] -> w829
              tunnel: [w846 w851] -> w824
              tunnel: w823 -> [w844 _]
              tunnel: w825 -> [_ w851]
              tunnel: w831 -> [w843 w850]
              tunnel: [w843 w850] -> w828
              tunnel: [w842 FALSE ("End")] -> w821
              frame No Error {
                n392 = call "SEND COMMAND TC-48-20.vi"("Communications Port"=w843, "Format String"="24%04x", "error in"=w847, "Data"=w844) -> ("CRC ERROR"=w846:bool, "End"=w842:bool, "error out"=w848:errorcluster)  [unwired: 1 in]
              }
              frame Error {
              }
            }
            n393 = case shown="No Error" w829 {
              selector: w829 -> [w837 w841]
              tunnel: w828 -> [w838 _]
              tunnel: [w836 w840] -> w827
              tunnel: [w835 w841] -> w826
              tunnel: w824 -> [_ w840]
              tunnel: [w833 FALSE ("End")] -> w820
              frame No Error {
                n394 = call "INPUT 1 SENSOR OFFSET M9613.vi"("Communications Port"=w838, "error in"=w837) -> ("CRC ERROR"=w836:bool, "End"=w833:bool, "INPUT 1 SENSOR OFFSET"=w834:dbl, "error out"=w835:errorcluster)
                n395 = property on="Control Sensor Offset" class="DigNum (strict)"("Value"=w834) -> ()  [unwired: 2 in, 2 out]
              }
              frame Error {
              }
            }
            n396 = Or(x=w821, y=w820) -> (x .or. y?=w819:bool)
          }
          event "EEPROM Write Enable": Value Change {
            n397 = event-data() -> ("NewVal"=w864:bool)  [unwired: 1 in]
            n398 = Boolean To (0,1)(Boolean=w864) -> (0, 1=w865:i16)
            n399 = case shown="No Error" w856 {
              selector: w856 -> [w880 w885]
              tunnel: [w881 w885] -> w862
              tunnel: [w876 w884] -> w858
              tunnel: w865 -> [w878 _]
              tunnel: w861 -> [_ w884]
              tunnel: w863 -> [w877 w883]
              tunnel: [w877 w883] -> w860
              tunnel: [w875 FALSE ("End")] -> w855
              frame No Error {
                n400 = call "SEND COMMAND TC-48-20.vi"("Communications Port"=w877, "Format String"="31%04x", "error in"=w880, "Data"=w878) -> ("CRC ERROR"=w876:bool, "End"=w875:bool, "error out"=w881:errorcluster)  [unwired: 1 in]
              }
              frame Error {
              }
            }
            n401 = case shown="No Error" w862 {
              selector: w862 -> [w870 w874]
              tunnel: w860 -> [w871 _]
              tunnel: [w869 w874] -> w859
              tunnel: w858 -> [_ w873]
              tunnel: [w867 w873] -> w857
              tunnel: [w866 FALSE ("End")] -> w853
              frame No Error {
                n402 = call "QUERY EEPROM WRITE ENABLE.vi"("Communications Port"=w871, "error IO"=w870) -> ("EEPROM WRITE\nENABLED"=w868:bool, "End"=w866:bool, "CRC"=w867:bool, "error IO 2"=w869:errorcluster)
                n403 = property on="EEPROM Write Enable" class="Bool (strict)"("Value"=w868) -> ()  [unwired: 2 in, 2 out]
              }
              frame Error {
              }
            }
            n404 = Or(x=w855, y=w853) -> (x .or. y?=w854:bool)
          }
          event Timeout {
            n405 = event-data() -> ()  [unwired: 1 in, 1 out]
          }
        }
      }
      frame Error {
      }
    }
    n406 = case shown="True" w72 {
      selector: w72 -> [_ w104]
      tunnel: [w101 w102] -> _
      tunnel: [w101 w103] -> w68
      tunnel: w71 -> [w101 w102]
      frame False {
      }
      frame True {
        n407 = Bundle By Name(cluster=w102, "CRC Error"=w104) -> (w103:T5)
      }
    }
    n408 = case shown="True" w66 {
      selector: w66 -> [_ w99]
      tunnel: w68 -> [w97 w100]
      tunnel: [w97 w98] -> w67
      frame False {
      }
      frame True {
        n409 = Bundle By Name(cluster=w100, "End"=w99) -> (w98:T5)
      }
    }
    n410 = case shown="Error" w84 {
      selector: w84 -> [w137 w139]
      tunnel: w67 -> [w138 w142]
      tunnel: [w138 w141] -> w70
      tunnel: [w137 w139] -> w79
      frame No Error {
      }
      frame Error {
        n411 = Two Button Dialog(message=" Unable to communicate with controller (Error 3), check:\n• Controller is ON and correctly wired\n• Correct communications port is selected\n• Another program is not using the communications port ", 1:"EXIT" ("F button name (\"Cancel\")"), 2:"RESTART" ("T button name (\"OK\")")) -> (T button?=w140:bool)
        n412 = case shown="True" w140 {
          selector: w140 -> [w148 _]
          tunnel: w142 -> [w146 w150]
          tunnel: [w147 w152] -> w141
          frame False {
            n413 = Not(x=w148) -> (.not. x?=w149:bool)
            n414 = Bundle By Name(cluster=w146, "End"=w149) -> (w147:T5)
          }
          frame True {
            w151 = TRUE
            n415 = Bundle By Name(cluster=w150, "Read Model"=w151, "Read Settings"=w151) -> (w152:T5)
          }
        }
      }
    }
    "error out" <- w79
    n416 = Unbundle By Name(w70) -> ("CRC Error"=w69:bool)
    "CRC Error" <- w69
    n417 = case shown="True" w69 {
      tunnel: [w1149 w1154] -> w64
      tunnel: w70 -> [w1149 w1155]
      frame False {
      }
      frame True {
        n418 = Two Button Dialog(message="COMMUNICATIONS\nERROR, CONTINUE?", 1:"STOP", 2:"CONTINUE") -> (T button?=w1150:bool)
        n419 = case shown="True" w1150 {
          selector: w1150 -> [w1158 _]
          tunnel: w1155 -> [w1156 w1160]
          tunnel: [w1157 w1162] -> w1154
          frame False {
            n420 = Not(x=w1158) -> (.not. x?=w1159:bool)
            n421 = Bundle By Name(cluster=w1156, "End"=w1159) -> (w1157:T5)
          }
          frame True {
            w1161 = TRUE
            n422 = Bundle By Name(cluster=w1160, "Read Model"=w1161, "Read Settings"=w1161) -> (w1162:T5)
          }
        }
      }
    }
    n423 = Unbundle By Name(w64) -> ("End"=w62:bool, "Final Loop"=w61:bool)
    n424 = And(x=w62, y=w61) -> (x .and. y?=w63:bool)
  }
